vi "Periodic Tasks.vi"(8 "error in":errorcluster) -> ()   [LabVIEW 2017]
doc: "This VI runs in parallel to other tasks. It can contain as many user-defined periodic loops as you need. These can carry out PID or other sorts of timed response."
uses:
  <vilib>/Rock Robotics/WPI/ThirdParty/Phoenix-LabVIEW/Motor Controller/Controls/CTRE_Phoenix_MotorControl_FeedbackDevice.ctl
  CommandTypes/DriveCommands.ctl
  <userlib>/836-Library/Drive/Drive_Code_V2/Drive_Code_Support/PidClusters/Drive_Code_PID_Bundle.ctl
  <vilib>/Platform/TimedLoop/XDataNode/timing_clust.ctl
  <vilib>/Platform/TimedLoop/XDataNode/nitl_modes.ctl
  <vilib>/Platform/TimedLoop/XDataNode/wakeup.ctl
  <userlib>/836-Library/Drive/Drive_Code_V2/Drive_Code_Support/SensorTypedefs/Sensor_Cluster.ctl
  <userlib>/836-Library/Drive/Drive_Code_V2/Drive_Code_Support/SensorTypedefs/Camera_Cluster.ctl
  <vilib>/Rock Robotics/WPI/RobotDrive/WPI_RobotDriveDevRef.ctl
  <vilib>/Rock Robotics/WPI/MotorControl/WPI_MotorControlDeviceRef.ctl
  <vilib>/Rock Robotics/WPI/MotorControl/WPI_MotorControlType.ctl
  <vilib>/Rock Robotics/SystemInterfaces/DIO/FPGA_DIOPWMChannel.ctl
  <vilib>/Rock Robotics/WPI/PWM/WPI_PWMDeadband.ctl
  <vilib>/Rock Robotics/SystemInterfaces/DIO/FPGA_DIOChannel.ctl
  <userlib>/836-Library/Drive/Drive_Code_V2/Drive_Code_Support/DriveTrains/Drive_Trains.ctl
  <userlib>/836-Library/Drive/Drive_Code_V2/Drive_Code_Support/Command_Sends/Drive_Code_Command_Type.ctl
  <userlib>/836-Library/Drive/Drive_Code_V2/Drive_Code_Support/Command_Sends/Drive_Code_Command_List.ctl
  <userlib>/836-Library/Drive/Drive_Code_V2/Drive_Code_Support/PidClusters/PidInversions.ctl
  <userlib>/836-Library/Drive/Drive_Code_V2/Drive_Code_Support/PidClusters/DrivePidInputs.ctl
  <userlib>/836-Library/Drive/Drive_Code_V2/Drive_Code_Support/PidClusters/PidInputs.ctl
  <userlib>/836-Library/Drive/Drive_Code_V2/Drive_Code_Support/Command_Sends/Command_Tolerances.ctl
  <userlib>/836-Library/Drive/Drive_Code_V2/Drive_Code_Support/Command_Sends/Command_Tolerance_Info.ctl
  <userlib>/836-Library/System/QCP_V2/QCPSupportCode/QCPData.ctl
  <vilib>/Rock Robotics/WPI/Relay/WPI_RelayValue.ctl
  <vilib>/Rock Robotics/WPI/DriverStation/WPI_DriverStationRobotMode2.ctl
  <userlib>/836-Library/Drive/Drive_Code_V2/Drive_Code_Support/CmdFinishedTypes.ctl
  <vilib>/Rock Robotics/WPI/ThirdParty/Phoenix-LabVIEW/Motor Controller/Get/CTRE_Phoenix_MotorController_GetPulseWidthAll.vi
  <vilib>/Rock Robotics/Network Tables/NT Read Number.vi
  <vilib>/Rock Robotics/Network Tables/NT Write Number.vi
  <userlib>/836-Library/Drive/Drive_Code_V2/Drive_Code_Support/Command_Sends/Drive_Cmd_PID_Update.vi
  <userlib>/836-Library/Drive/Drive_Code_V2/Drive_Code_Support/Command_Sends/Drive_Cmd_Follow_Camera.vi
  <userlib>/836-Library/Drive/Drive_Code_V2/Drive_Code_Support/Command_Sends/Drive_Cmd_Turn_to_Camera.vi
  <vilib>/addons/control/pid/pid.llb/PID Output Rate Limiter (DBL).vi
  <userlib>/836-Library/Drive/Drive_Code_V2/Drive_Code_Support/Command_Sends/Drive_Cmd_Cheesey_Drive.vi
  <vilib>/platform/TimedLoop/XDataNode/XDataNode.xnode
  <vilib>/Platform/TimedLoop/XDataNode/XDNodeRunTimeDep.lvlib
  <vilib>/addons/control/pid/NI_PID_pid.lvlib
  <vilib>/Rock Robotics/WPI/Power/WPI_Power Get 5Volt Rail Voltage and Current.vi
panel:
  in  "Tab Control":T1(tab)=enum."Sensors"
  out "SensorsFinished Late? [i-1]":bool=TRUE
  out "SensorsIterationDuration":i64=26
  out "QCP Finished Late? [i-1]":bool
  out "QCP Iteration Duration":i64=3
  in  "SensorPeriod":i64=20
  in  "QCPPeriod":i64=20
  out "DriveFinished Late? [i-1]":bool
  out "Drive Iteration Duration":i64=4
  in  "Drive Period":i64=40
  out "PID Finished Late? [i-1]":bool
  out "PID Iteration Duration":i64
  in  "PIDPeriod":i64=400
  out "Intake Iteration Duration":i64
  out "Intake Finished Late? [i-1]":bool
  in  "Intake Period":i64=50
  out "Lift Finished Late? [i-1]":bool=TRUE
  out "Lift Iteration Duration":i64=25
  in  "Lift Period":i64=20
  out "Lift_Command":T2(ring)=enum."Home"
  in  "Verticle_Mech_Hi":dbl
  in  "Verticle_Mech_Low":dbl=24.1875
  in  "Verticle_Sensor_Low":dbl=587.0
  in  "Rotation_Mech_Low":dbl=90.0
  in  "Verticle_Sensor_Hi":dbl=26537.0
  in  "Rotation_Mech_Hi":dbl
  in  "Rotation_Sensor_Low":dbl=6193.0
  in  "Rotation_Sensor_Hi":dbl=894.0
  in  "Position":dbl(knob) scale=0.0..1.0
  in  "Intake Speed":dbl(knob)=0.7699909222498021 scale=0.0..1.0
  out "Intake_Command":T3(ring)
  in  "Cube? Fakeout":bool=TRUE
  out "Cube?":bool=TRUE
  out "Steer Fed Value":dbl(graph)
  out "Dist Resp":cluster{"Setpoint":dbl, "Process":dbl}(graph)
  out "Angle Resp":cluster{"Setpoint":dbl, "Process":dbl}(graph)
  in  "Steer Scale":dbl(knob)=0.500001840510888 scale=0.0..1.0
  in  "Turn In Place Deadband":dbl(knob)=0.12768422674403432 scale=0.0..0.4
  in  "Throttle Scale":dbl(knob)=1.0 scale=0.0..1.0
  in  "Square Wheel":bool=TRUE
  in  "Square Throttle":bool=TRUE
  in  "Update PID":bool
  in  "AquireSpeed":dbl(knob) scale=0.0..10.0
  in  "CenterOnCubeTolerance":dbl=0.5
  in  "CenterSpeed":dbl(knob) scale=0.0..1.0
  in  "Yaw_Holding_Still_PID_Gains":T4={"proportional gain (Kc)"=0.021, "integral time (Ti, min)"=0.0, "derivative time (Td, min)"=0.0} {"derivative time (Td, min)" format="%.3f"; "integral time (Ti, min)" format="%.3f"; "proportional gain (Kc)" format="%.3f"}
  in  "Distance_Holding_Still_PID_gains":T4={"proportional gain (Kc)"=0.025, "integral time (Ti, min)"=0.013, "derivative time (Td, min)"=0.003} {"derivative time (Td, min)" format="%.3f"; "integral time (Ti, min)" format="%.3f"; "proportional gain (Kc)" format="%.3f"}
  in  "Distance_Driving_Straight_PID_Gains":T4={"proportional gain (Kc)"=0.025, "integral time (Ti, min)"=0.0125, "derivative time (Td, min)"=0.0025} {"derivative time (Td, min)" format="%.3f"; "integral time (Ti, min)" format="%.3f"; "proportional gain (Kc)" format="%.3f"}
  in  "Yaw_Driving_Straight_PID_gains":T4={"proportional gain (Kc)"=0.021, "integral time (Ti, min)"=0.0, "derivative time (Td, min)"=0.0} {"derivative time (Td, min)" format="%.3f"; "integral time (Ti, min)" format="%.3f"; "proportional gain (Kc)" format="%.3f"}
  out "Drive Command":T5(ring)=enum."Manual"
  in  "Acceleration Throttle Rate Limit":dbl(knob)=208.87815423820334 scale=200.0..400.0
  in  "Acceleration Steer Rate Limit":dbl(knob)=1540.1240783536919 scale=50.0..5000.0
  in  "Throttle Slow Mode Mult":dbl(knob)=0.518053304835497 scale=0.0..1.0
  in  "Steer Slow Mode Mult":dbl(knob)=0.5622816498580822 scale=0.0..1.0
  in  "Deceleration Steer Rate Limit":dbl(knob)=1e+27 scale=50.0..1e+27
  in  "DecelerationThrottle Rate Limit":dbl(knob)=1498.2967839773426 scale=200.0..1500.0
  in  "Read Drive QCP":bool
  in  "Read Lift QCP":bool
  in  "Read Auto QCP":bool
  in  "Read Intake QCP":bool
  in  "Read Sensor QCP":bool
  in  "DriveWriteQCPFile":bool
  in  "DriveTuningMode?":bool=TRUE
  in  "LiftWriteQCPFile":bool
  in  "LiftTuningMode?":bool=TRUE
  in  "AutoWriteQCPFile":bool
  in  "AutoTuningMode?":bool
  in  "IntakeWriteQCPFile":bool
  in  "IntakeTuningMode?":bool=TRUE
  in  "SensorWriteQCPFile":bool
  in  "SensorTuningMode?":bool
  out "Right Encoder":dbl(graph)=1039.4189824999999
  out "Left Encoder":dbl(graph)
  in  "PBot Lift Pitch Ref":dbl=230.0
  in  "Reset Lift Rate":bool
  out "IMU Rate Lift":dbl
  out "IMU Lift Max Rate":dbl
  out "IMU LIft Rate":dbl(graph)
  in  "Lift Is IMU?":bool
  out "Pitch  Drive":dbl(graph)
  out "Roll Drive":dbl(graph)
  out "Yaw Drive":dbl(graph)
  out "RightDriveEncoder":dbl=1039.4189824999999
  out "Cube? 4":bool
  out "LeftDriveEncoder":dbl=801.3391574999999
  out "LiftElevation":dbl=-21.72307803468208
  out "LiftRotation":dbl=-14.878278920551049
  out "Cube? 3":bool
  out "Cube? 5":bool
  out "Cube? 6":bool
  out "Cube? 1":bool
  out "Cube? 2":bool
  out "Yaw Wind Drive":dbl
  out "Roll Wind Drive":dbl
  out "Pitch Wind Drive":dbl
  out "Valid Target":bool
  out "tx":dbl
  in  "ledMode":dbl=1.0
  in  "pipeline":dbl
  in  "userMode":dbl
  in  "Restart Limelight":bool
  out "Yaw Wind LiftArm":dbl
  out "Roll WindLiftArm":dbl
  out "Pitch LiftArm":dbl=-87.0
  out "YawLiftArm":dbl(graph)
  out "Roll LiftArm":dbl(graph)
  out "Pitch LiftArm":dbl(graph)
  out "Raw Lift Elevation":i32=3231
  out "Raw Lift Rotation":i32=1770
  in  "Lift Pitch Ref":dbl=87.0
  out "Lift IMU Fault":bool
  in  "Hyster":dbl=0.3
  in  "Rate Thresh":dbl=500.0 step=0.001
  in  "hi limit":dbl=35.0
  in  "lo limit":dbl=-211.0
  out "Total Current (A)":dbl
  out "Current (A)":dbl
  in  "Reet Max Total":bool
  out "Max Total Current":dbl=282.75
  out "PDP Total Current":dbl(graph)
  in  "Reset Max Current?":bool
  out "Max Current (A)":dbl
  in  "PDP Channel":dbl=10.0
  out "PDP Channel Current (A)":dbl(graph)
  out "Input Voltage Brown Out":bool
  out "3.3V User Rail Short":bool
  out "5 V User Rail Short":bool
  out "6 V User Rail Short":bool
  out "5V User Rail Brown Out":bool
  out "5 volt rail voltage (V)":dbl=4.950481445312501
  out "5 volt rail current (A)":dbl=0.289408203125
  in  "Reset Voltage Max":bool
  out "Voltage Min":dbl=4.949025878906251
  in  "Reset Current Max":bool
  out "5V Rail Current Max":dbl=0.289408203125
  in  "Current Tolerance":dbl=100.0
  in  "Current Limit?":bool=TRUE
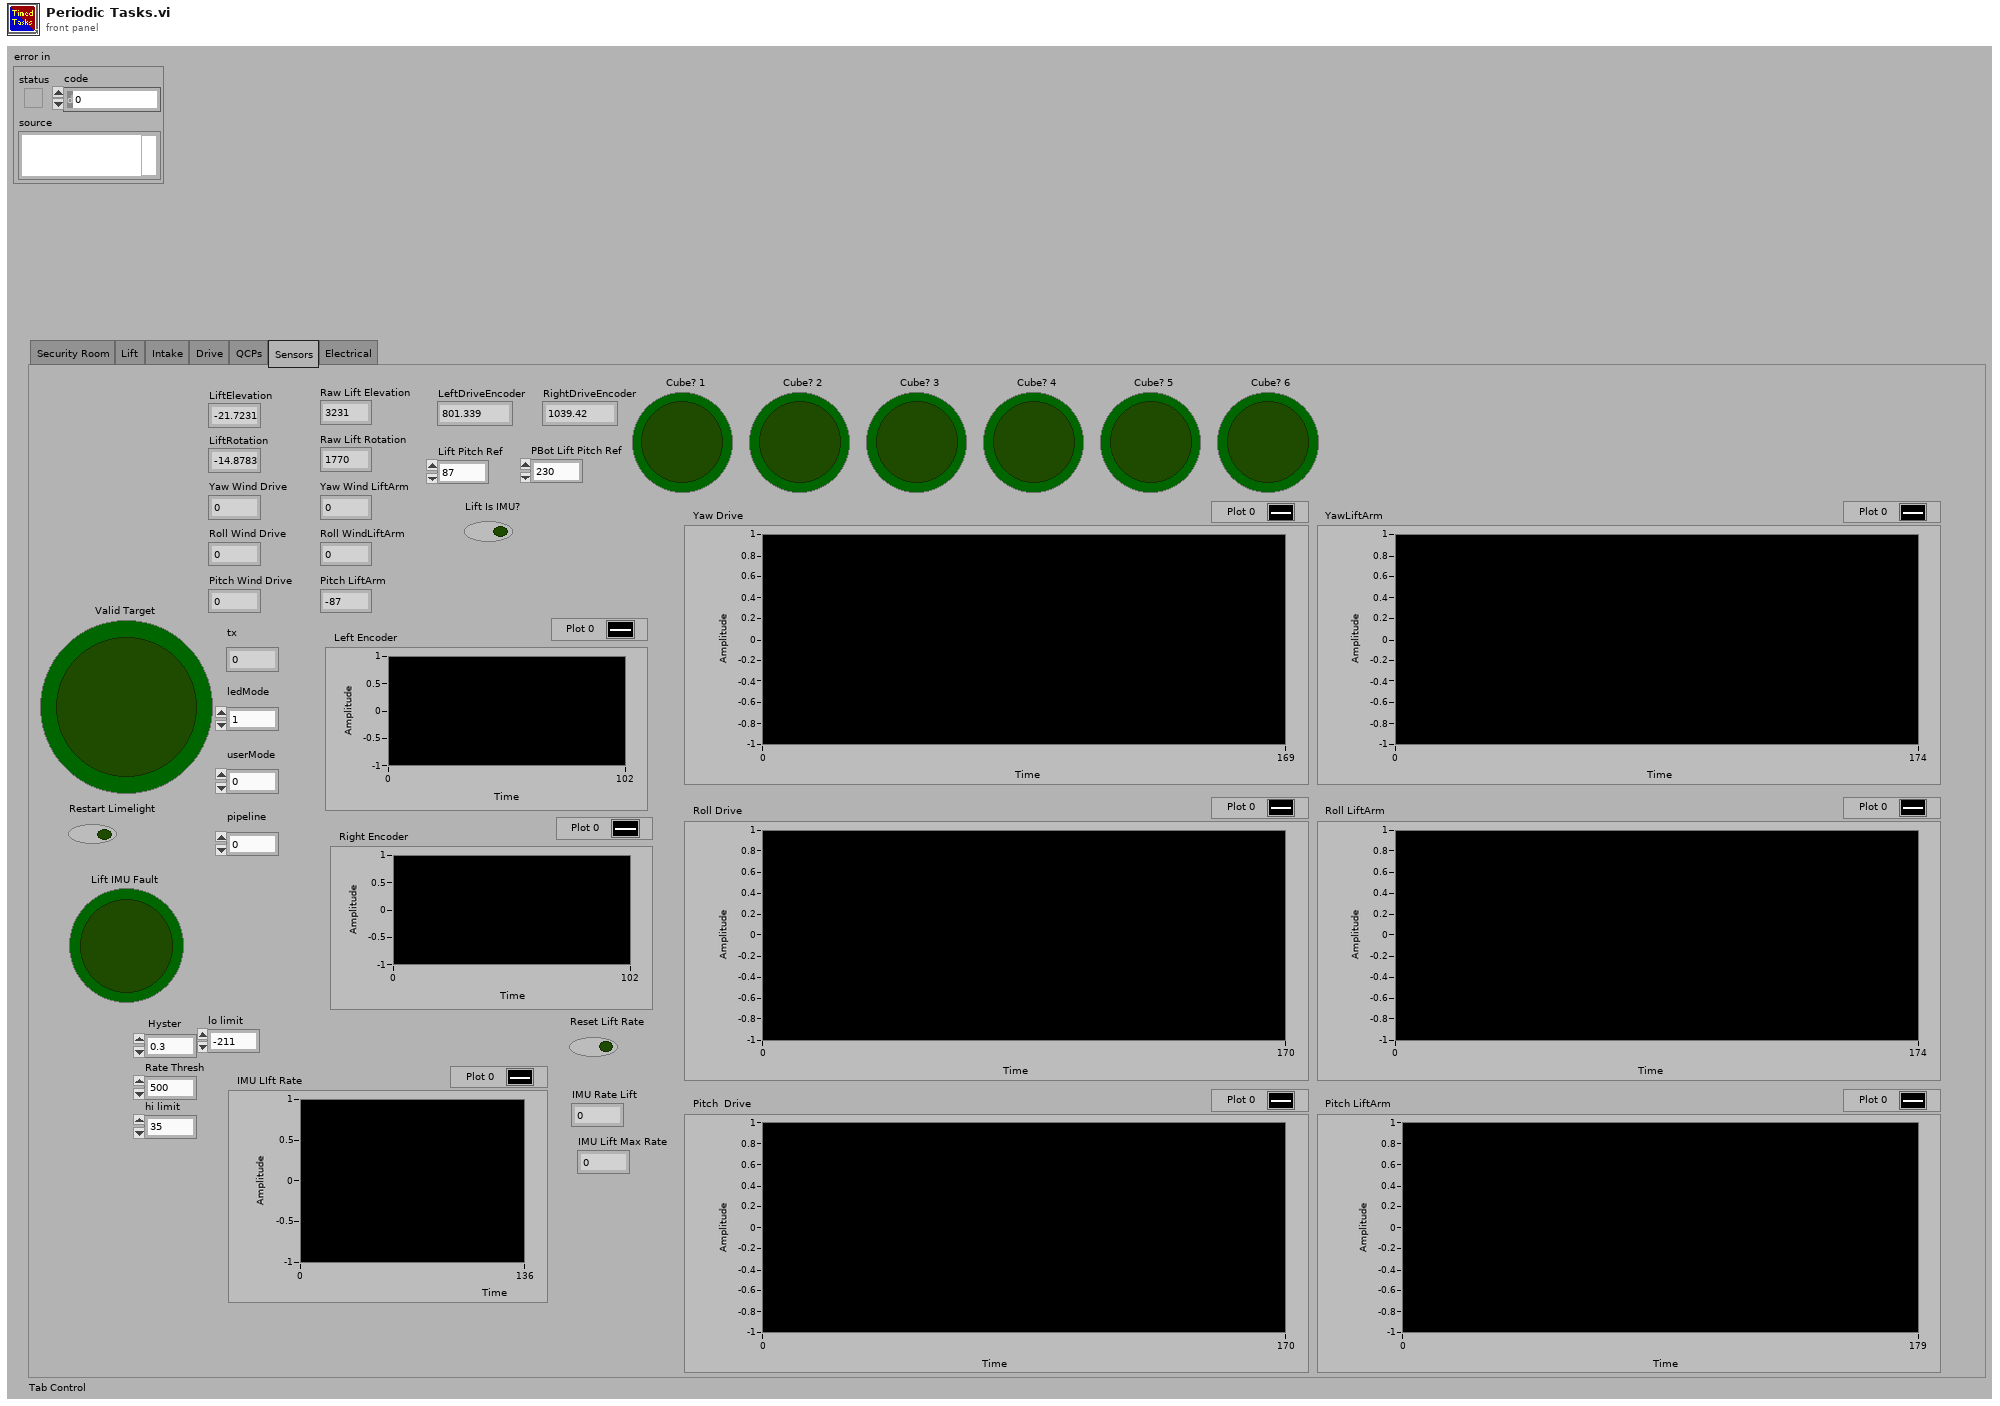
[diagram p1: front panel]
types:
  T1 = enum32{"Security Room", "Lift", "Intake", "Drive", "QCPs", "Sensors", "Electrical"}
  T2 = enum16{"Do  Nothing", "Manuel", "Home", "Ground", "To Switch", "To Scale Low", "To Scale Medium", "To Scale High"}
  T3 = enum16{"Do Nothing", "Manuel", "Score", "Acquire"}
  T4 = cluster{"proportional gain (Kc)":dbl, "integral time (Ti, min)":dbl, "derivative time (Td, min)":dbl}
  T5 = enum16{"Center on Cube", "Manual", "Acquire Cube", "Drive Path"}
  T6 = typedef "Drive_Code_PID_Bundle.ctl" = cluster{"Yaw, Driving Straight":cluster{"proportional gain (Kc)":dbl, "integral time (Ti, min)":dbl, "derivative time (Td, min)":dbl}, "Yaw, Holding Still":cluster{"proportional gain (Kc)":dbl, "integral time (Ti, min)":dbl, "derivative time (Td, min)":dbl}, "Distance, Driving Straight":cluster{"proportional gain (Kc)":dbl, "integral time (Ti, min)":dbl, "derivative time (Td, min)":dbl}, "Distance, Holding Still":cluster{"proportional gain (Kc)":dbl, "integral time (Ti, min)":dbl, "derivative time (Td, min)":dbl}}
  T7 = typedef "DriveCommands.ctl" = enum16{"Center on Cube", "Manual", "Acquire Cube", "Drive Path"}
  T8 = typedef "CTRE_Phoenix_MotorControl_FeedbackDevice.ctl" = i8
  T9 = typedef "WPI_MotorControlDeviceRef.ctl" = cluster{"DeviceStatus":errorcluster, "Type":T10, "PWM":cluster{"PWM Channel":T11, "DeadBand":T12}, "CAN":cluster{"Device Number":u8, "SetOutput VI Ref":variant, "GetOutput VI Ref":variant, "Enable VI Ref":variant, "Disable VI Ref":variant, "Data":variant}, "Invert":bool, "DIO PWM":cluster{"PWM \"Enable\" Channel":T11, "DIOChannel":T13, "PWM Rate":dbl}}
  T10 = typedef "WPI_MotorControlType.ctl" = enum16{"PWM", "CAN", "DIO PWM"}
  T11 = typedef "FPGA_DIOPWMChannel.ctl" = enum8{"PWM 0", "PWM 1", "PWM 2", "PWM 3", "PWM 4", "PWM 5", "PWM 6", "PWM 7", "PWM 8", "PWM 9", "PWM MXP 0", "PWM MXP 1", "PWM MXP 2", "PWM MXP 3", "PWM MXP 4", "PWM MXP 5", "PWM MXP 6", "PWM MXP 7", "PWM MXP 8", "PWM MXP 9", "Invalid"}
  T12 = typedef "WPI_PWMDeadband.ctl" = cluster{"Name":string, "maxPositivePwm":i32, "minPositivePwm":i32, "centerPwm":i32, "maxNegativePwm":i32, "minNegativePwm":i32, "angularRange":u16}
  T13 = typedef "FPGA_DIOChannel.ctl" = enum8{"DIO 0", "DIO 1", "DIO 2", "DIO 3", "DIO 4", "DIO 5", "DIO 6", "DIO 7", "DIO 8", "DIO 9", "DIO MXP 0", "DIO MXP 1", "DIO MXP 2", "DIO MXP 3", "DIO MXP 4", "DIO MXP 5", "DIO MXP 6", "DIO MXP 7", "DIO MXP 8", "DIO MXP 9", "DIO MXP 10", "DIO MXP 11", "DIO MXP 12", "DIO MXP 13", "DIO MXP 14", "DIO MXP 15", "SPI Port CS1", "SPI Port CS2", "SPI Port CS3", "SPI Port MISO", "SPI Port MOSI", "Invalid"}
  T14 = typedef "WPI_DigitalInputDevRef.ctl" = cluster{"DevStatus":errorcluster, "DIO Channel":T13}
  T15 = typedef "XDNodeRunTimeDep.lvlib/timing_clust.ctl" = cluster{"Expected End [f-1]":u64, "Actual End [f-1]":u64, "Finished Late? [f-1]":bool, "Expected End [i-1]":u64, "Actual End [i-1]":u64, "Finished Late? [i-1]":bool, "Expected Start [i]":u64, "Actual Start [i]":u64, "Expected Start [f]":u64, "Actual Start [f]":u64, "Source Name":string, "Structure Name":string, "Period":i64, "Deadline":i64, "Offset":i64, "Start":i64, "Priority":i32, "Timeout":i32, "Mode":T16, "Wakeup Reason":T17, "Error":errorcluster, "Source Type":string, "Secondary Source Type":string, "Global End Time":u64, "Global Start Time":u64, "Frame Duration":u64, "Iteration Duration":u64, "Assigned CPU":i32, "I/O Scan Engine Mode":u32}
  T16 = typedef "XDNodeRunTimeDep.lvlib/nitl_modes.ctl" = enum32{"No Change", "Process missed periods, maintain original phase", "Discard missed periods, maintain original phase", "Process missed periods, ignore original phase", "Discard missed periods, ignore original phase"}
  T17 = typedef "XDNodeRunTimeDep.lvlib/wakeup.ctl" = enum32{"Normal", "Aborted", "Asynchronous wakeup", "Timing source error", "Timed loop error", "Timeout"}
  T18 = typedef "WPI_EncoderDevRef.ctl" = cluster{"DevStatus":errorcluster, "EncoderIndex":T19, "CounterIndex":T20, "DistancePerCount":dbl, "Decoding Type":T21}
  T19 = typedef "FPGA_EncoderIdx.ctl" = enum8{"Enc 0", "Enc 1", "Enc 2", "Enc 3", "Enc 4", "Enc 5", "Enc 6", "Enc 7", "Invalid"}
  T20 = typedef "FPGA_CounterCtrSystemIndex.ctl" = enum8{"Ctr 0", "Ctr 1", "Ctr 2", "Ctr 3", "Ctr 4", "Ctr 5", "Ctr 6", "Ctr 7", "Invalid"}
  T21 = typedef "WPI_EncoderType.ctl" = enum16{"1x", "2x", "4x"}
  T22 = typedef "ImuDevRef.ctl" = cluster{"I2CDevRef":T23, "Valid Cal File?":bool}
  T23 = typedef "WPI_I2CDevRef.ctl" = cluster{"DevStatus":errorcluster, "Device Address":u8, "Handle":i32, "I2C Bus":T24}
  T24 = typedef "i2c_bus.ctl" = enum16{"I2C On-Board", "I2C MXP", "Invalid"}
  T25 = typedef "WPI_RelayDevRef.ctl" = cluster{"DevStatus":errorcluster, "Relay Channel":T26, "Relay Direction":T27}
  T26 = typedef "FPGA_DIORelayChannel.ctl" = enum8{"Relay 0", "Relay 1", "Relay 2", "Relay 3", "Invalid"}
  T27 = typedef "WPI_RelayDirection.ctl" = enum16{"Both directions", "Forward only", "Reverse only"}
  T28 = typedef "WPI_RelayValue.ctl" = enum16{"Off", "On", "Forward", "Reverse"}
  T29 = enum16{"[0, 360]", "[-180, 180]", "[0, 2PI]", "[-PI, PI]"}
  T30 = cluster{"Yaw":dbl, "Roll":dbl, "Pitch":dbl, "Yaw Wind":dbl, "Roll Wind":dbl, "Pitch Wind":dbl}
  T31 = typedef "Sensor_Cluster.ctl" = cluster{"Gyro Data":cluster{"Gyro RT FIFO":refnum<k33>, "Gyro Current":dbl, "Gyro Hold":dbl}, "Encoder Data":cluster{"Encoder RT FIFO":refnum<k33>, "Encoder Current":dbl, "Encoder Hold":dbl}, "Camera Data":cluster{"Camera RT FIFO":refnum<k33>, "Camera Current":T32}}
  T32 = typedef "Camera_Cluster.ctl" = cluster{" Angle":dbl, "Valid":bool}
  T33 = typedef "WPI_RobotDriveDevRef.ctl" = cluster{"DevStatus":errorcluster, "Motors[]":T9[], "Square Inputs":bool, "Max Output":dbl}
  T34 = typedef "Drive_Trains.ctl" = enum16{"Tank Drive 2 Motor", "Tank Drive 4 Motor", "Tank Drive 6 Motor", "Mecanum Drive", "Kiwi Drive", "Invalid"}
  T35 = typedef "PidInversions.ctl" = cluster{"Distance PID Inverted?":bool, "Yaw PID Inverted?":bool}
  T36 = cluster{"Cluster":T31, "RobotDriveDevRef":T33, "Enum":T34, "Valid Commands":bool[], "Drive Comand Notifier":refnum<notifier>, "Command Finished?":refnum<k4>, "Command Canceled":refnum<k4>, "PID Inversions":T35, "PID Inputs Notifier":refnum<notifier>, "Cmd Tol Notifier":refnum<notifier>}
  T37 = typedef "Semaphore RefNum" = refnum<k1>
  T38 = cluster{"Data Value Refnum":refnum<data-value>, "semaphore":T37}
  T39 = typedef "QCP_RefNum.ctl" = cluster{"Data Value Refnum":refnum<data-value>, "semaphore":T37}
  T40 = typedef "WPI_ServoDeviceRef.ctl" = cluster{"DeviceStatus":errorcluster, "PWM Channel":T11, "DeadBand":T12}
  T41 = typedef "Command_Tolerances.ctl" = cluster{"Distance":T42, "Yaw":T42}
  T42 = typedef "Command_Tolerance_Info.ctl" = cluster{"Upper Error Bound":dbl, "Lower Error Bound":dbl}
  T43 = typedef "WPI_DriverStationRobotMode2.ctl" = enum16{"Autonomous Disabled", "Autonomous Enabled", "Teleop Disabled", "Teleop Enabled", "Disconnected", "Finish", "Test Disabled", "Test Enabled", "Emergency Stopped"}
  T44 = typedef "CmdFinishedTypes.ctl" = enum16{"Poll", "Blocking"}
  T45 = typedef "DrivePidInputs.ctl" = cluster{"EncoderPID":T46, "YawPID":T46}
  T46 = typedef "PidInputs.ctl" = cluster{"Setpoint":dbl, "Process":dbl}
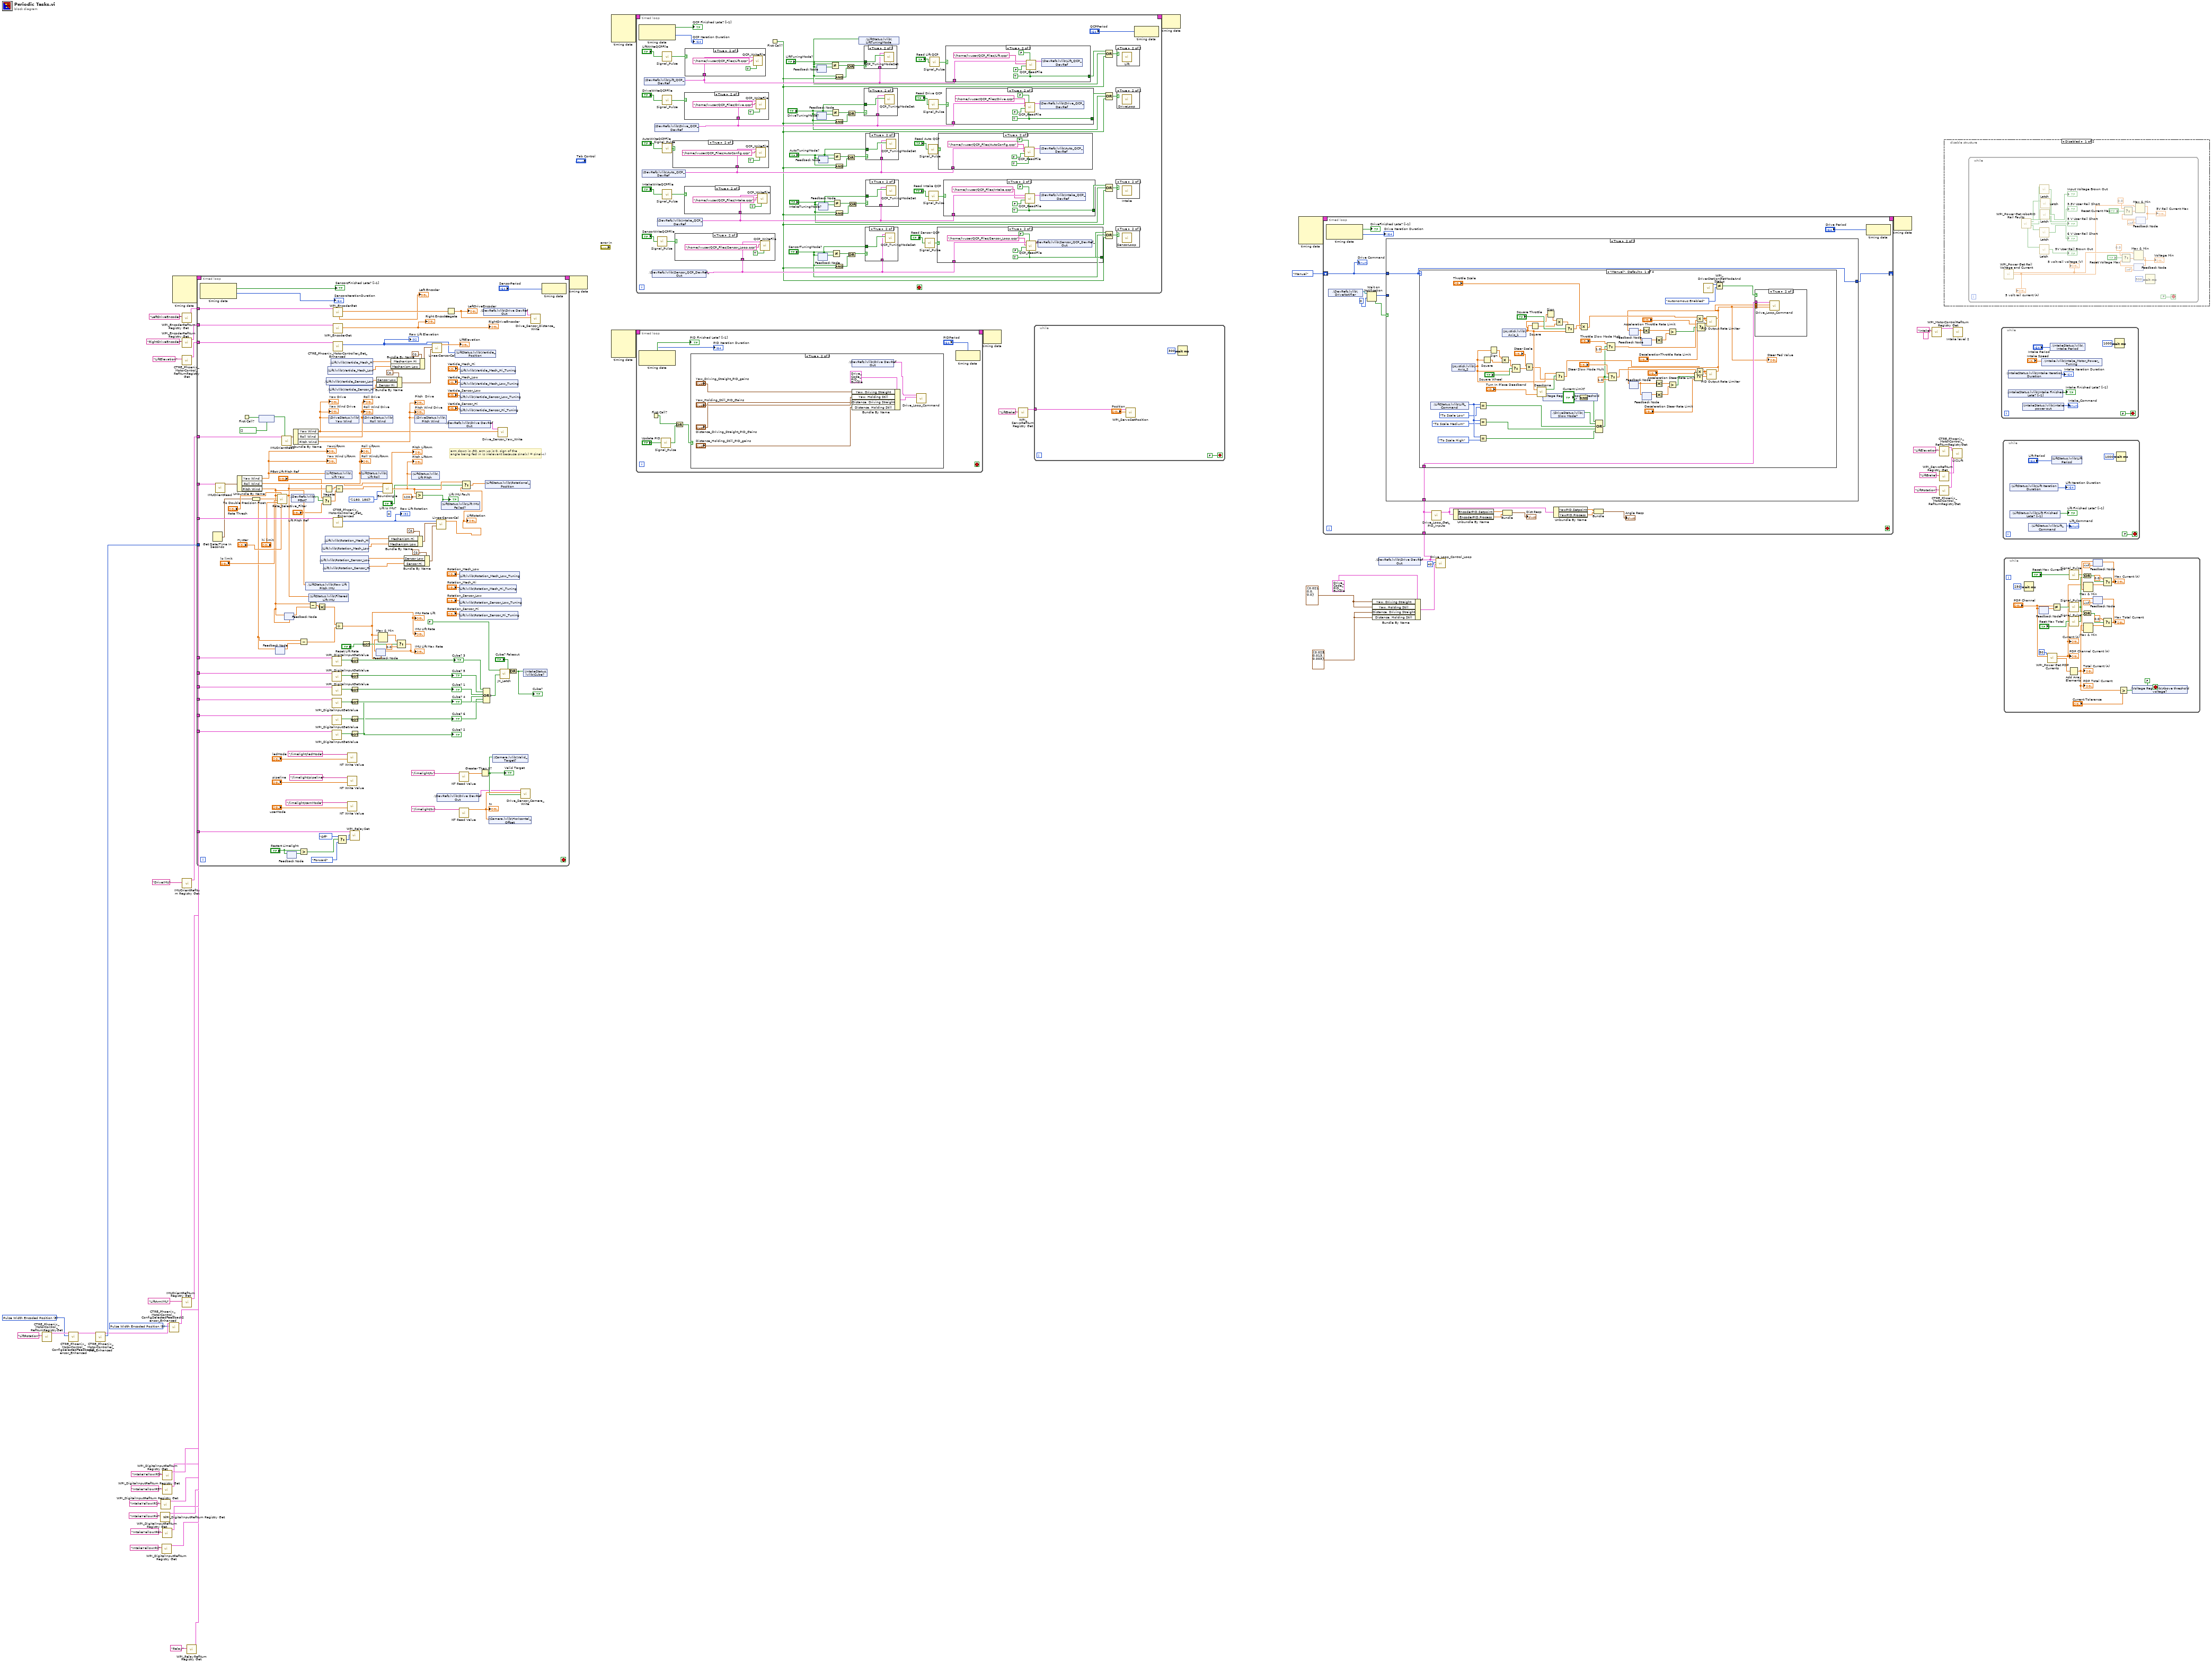
[diagram p0: block diagram]
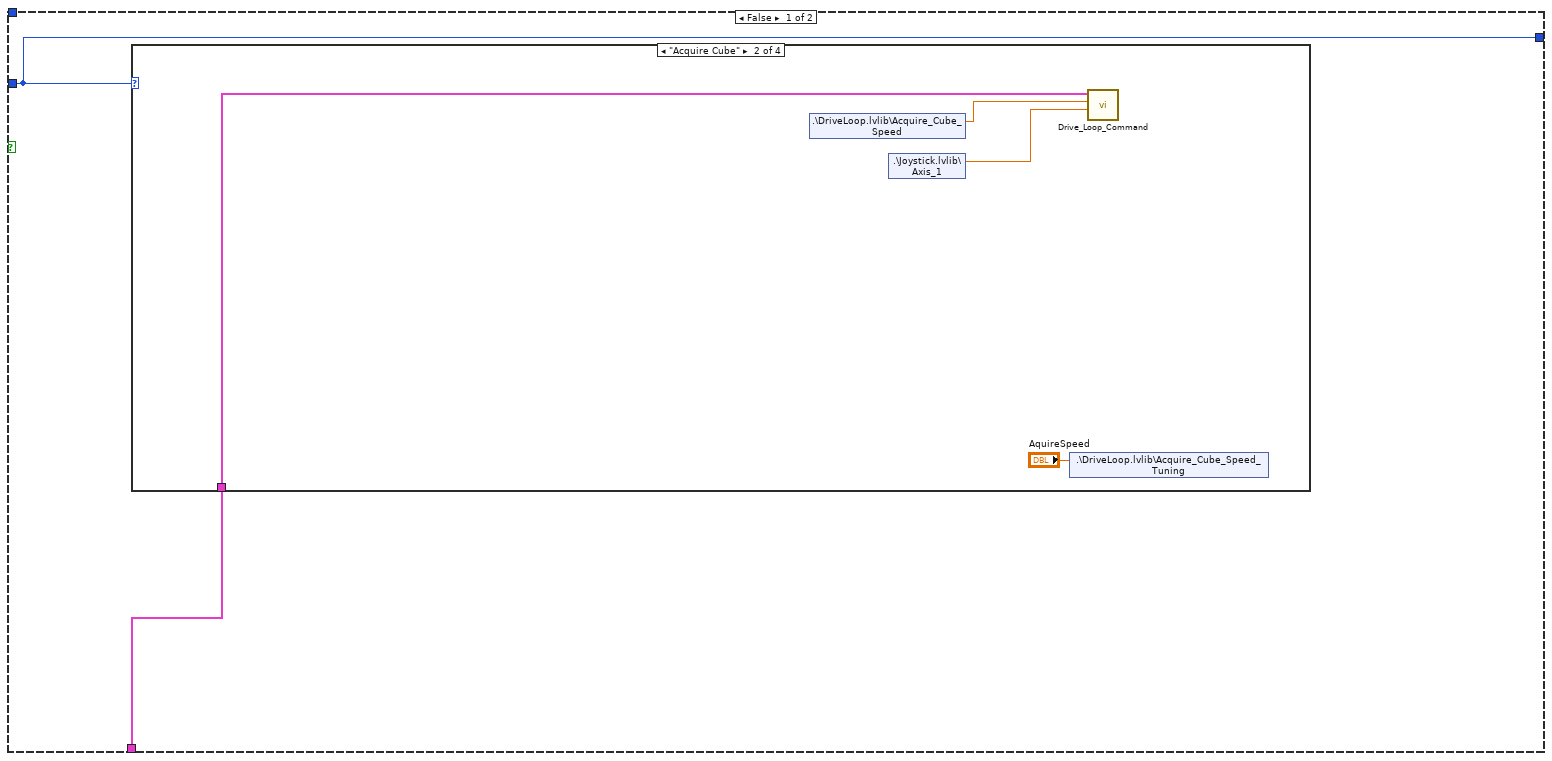
[diagram p2: hidden frame]
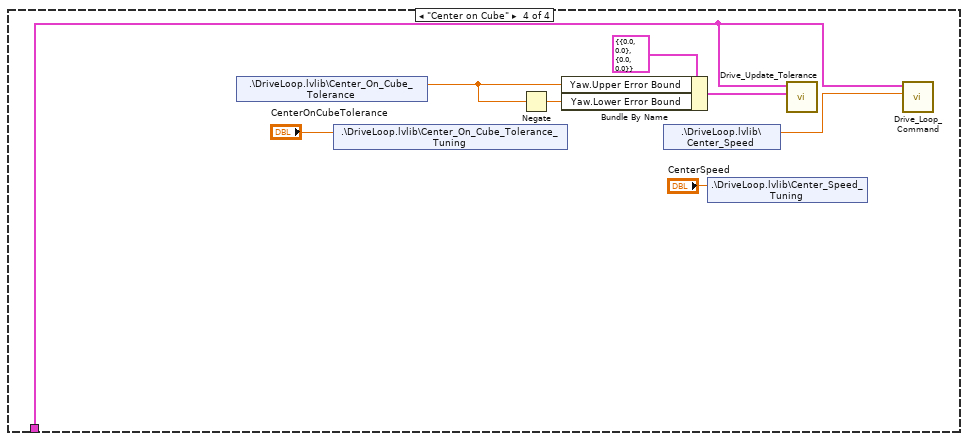
[diagram p5: hidden frame]
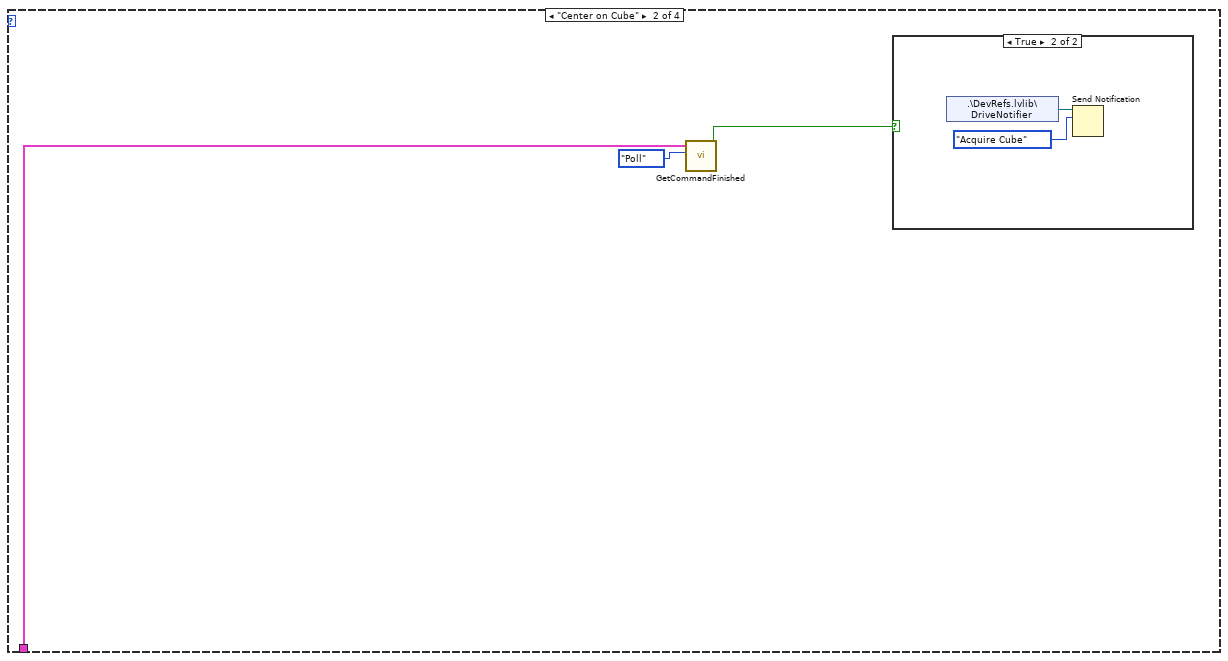
[diagram p7: hidden frame]
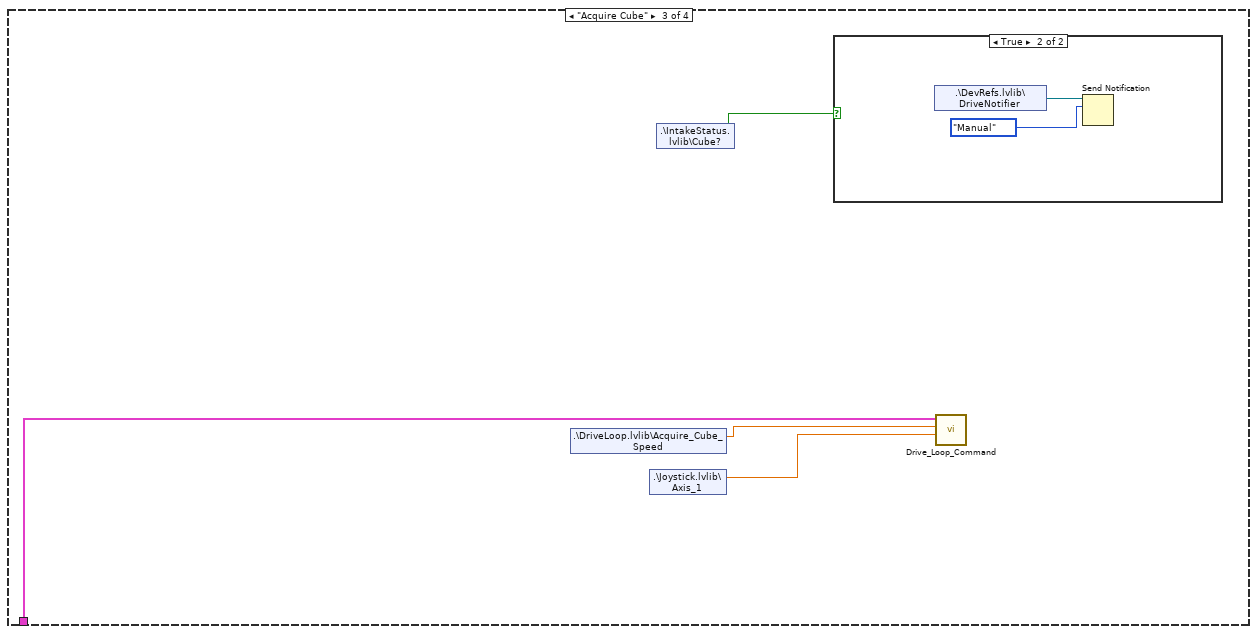
[diagram p9: hidden frame]
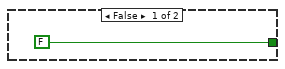
[diagram p17: hidden frame]
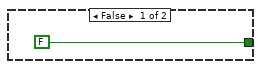
[diagram p18: hidden frame]
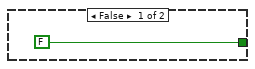
[diagram p20: hidden frame]
diagram:
  w4 = T4 {"proportional gain (Kc)"=0.025, "integral time (Ti, min)"=0.013, "derivative time (Td, min)"=0.003} ("Distance, Driving Straight")
  w5 = T4 {"proportional gain (Kc)"=0.021, "integral time (Ti, min)"=0.0, "derivative time (Td, min)"=0.0} ("Yaw, Driving Straight")
  w35 = T8 8 items=["None"=-1, "QuadEncoder"=0, "Analog"=2, "Tachometer"=4, "Pulse Width Encoded Position"=8, "Sensor Sum (S0 + S1)"=9, "Sensor Difference (D0 - D1)"=10, "Remote Source 0"=11, "Remote Source 1"=12, "Software Emulated"=15] ("Feedback Device")
  w39 = T8 8 items=["None"=-1, "QuadEncoder"=0, "Analog"=2, "Tachometer"=4, "Pulse Width Encoded Position"=8, "Sensor Sum (S0 + S1)"=9, "Sensor Difference (D0 - D1)"=10, "Remote Source 0"=11, "Remote Source 1"=12, "Software Emulated"=15] ("Feedback Device")
  n1 = call <vilib>:"CTRE_Phoenix_MotorControl_RefNumRegistryGet.vi"("refnum name"="LiftRotation") -> ("PhoenixMotorControlDevRef"=w40:T9)  [unwired: 9 in, 1 out]
  n2 = call <vilib>:"CTRE_Phoenix_MotorControl_ConfigSelectedFeedbackSensor_Enhanced.vi"("Feedback Device"=w39, "PhoenixMotorControlDevRef"=w40) -> ("PhoenixMotorControlDevRef"=w38:T9)  [unwired: 8 in, 1 out]
  n3 = call-poly <vilib>:"CTRE_Phoenix_MotorController_Get_Enhanced.vi"("PhoenixMotorControlDevRef"=w38) -> ("PhoenixMotorControlDevRef"=w36:T9, "Pulse Width Position"=w37:i32)  [unwired: 9 in, 4 out]
  n4 = call <vilib>:"WPI_DigitalInputRefNum Registry Get.vi"("refnum name"="IntakeYellowIR4") -> ("DigitalInputDevRef"=w55:T14)  [unwired: 9 in, 1 out]
  n5 = call <vilib>:"WPI_DigitalInputRefNum Registry Get.vi"("refnum name"="IntakeYellowIR1") -> ("DigitalInputDevRef"=w46:T14)  [unwired: 9 in, 1 out]
  n6 = call <vilib>:"WPI_DigitalInputRefNum Registry Get.vi"("refnum name"="IntakeYellowIR2") -> ("DigitalInputDevRef"=w45:T14)  [unwired: 9 in, 1 out]
  n7 = call <vilib>:"WPI_DigitalInputRefNum Registry Get.vi"("refnum name"="IntakeYellowIR5") -> ("DigitalInputDevRef"=w48:T14)  [unwired: 9 in, 1 out]
  n8 = call <vilib>:"WPI_DigitalInputRefNum Registry Get.vi"("refnum name"="IntakeYellowIR6") -> ("DigitalInputDevRef"=w47:T14)  [unwired: 9 in, 1 out]
  n9 = call <vilib>:"WPI_DigitalInputRefNum Registry Get.vi"("refnum name"="IntakeYellowIR3") -> ("DigitalInputDevRef"=w53:T14)  [unwired: 9 in, 1 out]
  n10 = call <vilib>:"CTRE_Phoenix_MotorControl_ConfigSelectedFeedbackSensor_Enhanced.vi"("Feedback Device"=w35, "PhoenixMotorControlDevRef"=w36) -> ("PhoenixMotorControlDevRef"=w34:T9)  [unwired: 8 in, 1 out]
  n11 = node-c288() -> (w31:T15)  [unwired: 4 in]
  n12 = call <vilib>:"WPI_EncoderRefNum Registry Get.vi"("refnum name"="LeftDriveEncoder") -> ("EncoderDevRef"=w22:T18)  [unwired: 9 in, 1 out]
  n13 = call <vilib>:"WPI_EncoderRefNum Registry Get.vi"("refnum name"="RightDriveEncoder") -> ("EncoderDevRef"=w23:T18)  [unwired: 9 in, 1 out]
  n14 = call <vilib>:"CTRE_Phoenix_MotorControl_RefNumRegistryGet.vi"("refnum name"="LiftElevation") -> ("PhoenixMotorControlDevRef"=w24:T9)  [unwired: 9 in, 1 out]
  n15 = call <userlib>:"IMUOrientRefNum Registry Get.vi"("refnum name"="DriveIMU") -> ("IMUDevRef out"=w28:T22)  [unwired: 9 in, 1 out]
  n16 = call <userlib>:"IMUOrientRefNum Registry Get.vi"("refnum name"="LiftArmIMU") -> ("IMUDevRef out"=w41:T22)  [unwired: 9 in, 1 out]
  n17 = call <vilib>:"WPI_RelayRefNum Registry Get.vi"("refnum name"="Relay") -> ("RelayDevRef"=w43:T25)  [unwired: 9 in, 1 out]
  n18 = timed-loop {
    timing: w31 -> [_]
    timing-out: [_] -> w30
    tunnel: w55 -> [w184]
    tunnel: w34 -> [w183]
    tunnel: w24 -> [w182]
    tunnel: w23 -> [w181]
    tunnel: w22 -> [w180]
    tunnel: w28 -> [w176]
    tunnel: w53 -> [w174]
    tunnel: w48 -> [w173]
    tunnel: w47 -> [w172]
    tunnel: w46 -> [w171]
    tunnel: w45 -> [w170]
    tunnel: w43 -> [w135]
    tunnel: w41 -> [w128]
    tunnel: w37 -> [_]
    stop <- _ stop-if-true
    (unwired) 0
    # "arm down is -90, arm up is 0. sign of the \nangle being fed in is irrelevant because sine(x) = sine(-x)"
    n19 = node-c288() -> (→"SensorsFinished Late? [i-1]":bool, →"SensorsIterationDuration":i64)  [unwired: 1 in]
    n20 = Get Date/Time In Seconds() -> (seconds since 1Jan1904=w79:timestamp)
    n21 = call <userlib>:"IMUOrientRead.vi"("IMU Dev Ref"=w128) -> ("Orient Y/R/P"=w127:T30)  [unwired: 7 in, 7 out]
    n22 = Unbundle By Name(w127) -> ("Yaw Wind"=w130:dbl, "Roll Wind"=w129:dbl, "Pitch Wind"=w77:dbl)
    "Yaw Wind LiftArm" <- w130
    "Roll WindLiftArm" <- w129
    "YawLiftArm" <- w130
    "Roll LiftArm" <- w129
    n23 = First Call?() -> (First Call?: T/F=w125:bool)
    n24 = To Double Precision Float(number=w79) -> (double precision float=w69:dbl)
    n25 = feedback #1(bool[] []) -> (w124:bool)
    n26 = feedback-in #1(w125) -> ()
    n27 = feedback-in #2(w69) -> ()
    n28 = feedback #2() -> (w68:dbl)  [unwired: 1 in]
    n29 = call <userlib>:"Rate_Selective_Filter.vi"("Hyster"="Hyster", "Rate Thresh"="Rate Thresh", "hi limit"="hi limit", "lo limit"="lo limit", "Time"=w69, "Distance"=w77) -> ("Filtered"=w80:dbl)  [unwired: 1 in, 2 out]
    "Pitch LiftArm" <- w80
    n30 = call <userlib>:"IMUOrientRead.vi"("IMU Dev Ref"=w176, "Orient Reset (Wind)"=w124) -> ("Orient Y/R/P"=w175:T30)  [unwired: 6 in, 7 out]
    n31 = feedback-in #3(w77) -> ()
    n32 = feedback #3(w77) -> (w78:dbl)
    n33 = feedback #4() -> (w89:bool)  [unwired: 1 in]
    n34 = feedback-in #4("Restart Limelight") -> ()
    n35 = shared-variable ".\\DevRefs.lvlib\\PBot?"() -> (w61:bool)  [unwired: 1 in, 1 out]
    n36 = Unbundle By Name(w175) -> ("Yaw Wind"=w115:dbl, "Roll Wind"=w154:dbl, "Pitch Wind"=w153:dbl)
    "Yaw Wind Drive" <- w115
    "Roll Wind Drive" <- w154
    "Pitch Wind Drive" <- w153
    "Yaw Drive" <- w115
    "Roll Drive" <- w154
    "Pitch  Drive" <- w153
    n37 = Subtract(x=w69, y=w68) -> (x-y=w66:dbl)
    n38 = Greater?(x="Restart Limelight", y=w89) -> (0:w90:bool)
    n39 = shared-variable ".\\LiftStatus.lvlib\\Raw Lift Pitch IMU"(w77) -> ()  [unwired: 1 in, 1 out]
    n40 = Subtract(x=w77, y=w78) -> (x-y=w76:dbl)
    n41 = shared-variable ".\\LiftStatus.lvlib\\Filtered Lift IMU"(w80) -> ()  [unwired: 1 in, 1 out]
    n42 = Absolute Value(x=w76) -> (abs(x)=w67:dbl)
    n43 = shared-variable ".\\Lift.lvlib\\Rotation_Sensor_Low"() -> (w148:dbl)  [unwired: 1 in, 1 out]
    n44 = Select(t="PBot Lift Pitch Ref", s=w61, f="Lift Pitch Ref") -> (s? t:f=w64:dbl)
    n45 = shared-variable ".\\Lift.lvlib\\Rotation_Mech_Low"() -> (w163:dbl)  [unwired: 1 in, 1 out]
    n46 = shared-variable ".\\Lift.lvlib\\Rotation_Sensor_Hi"() -> (w147:dbl)  [unwired: 1 in, 1 out]
    n47 = Negate(x=w80) -> (-x=w123:dbl)
    n48 = shared-variable ".\\LiftStatus.lvlib\\Lift Yaw"(w130) -> ()  [unwired: 1 in, 1 out]
    n49 = shared-variable ".\\Lift.lvlib\\Rotation_Mech_Hi"() -> (w149:dbl)  [unwired: 1 in, 1 out]
    n50 = shared-variable ".\\Lift.lvlib\\Verticle_Sensor_Low"() -> (w140:dbl)  [unwired: 1 in, 1 out]
    n51 = shared-variable ".\\Lift.lvlib\\Verticle_Mech_Low"() -> (w141:dbl)  [unwired: 1 in, 1 out]
    n52 = shared-variable ".\\DriveStatus.lvlib\\Yaw Wind"(w115) -> ()  [unwired: 1 in, 1 out]
    n53 = shared-variable ".\\Lift.lvlib\\Verticle_Sensor_Hi"() -> (w139:dbl)  [unwired: 1 in, 1 out]
    n54 = shared-variable ".\\Lift.lvlib\\Verticle_Mech_Hi"() -> (w138:dbl)  [unwired: 1 in, 1 out]
    n55 = call <vilib>:"WPI_DigitalInputGetValue.vi"("DigitalInputDevRef"=w174) -> ("Value"=w169:bool)  [unwired: 8 in, 2 out]
    n56 = call <vilib>:"WPI_DigitalInputGetValue.vi"("DigitalInputDevRef"=w173) -> ("Value"=w168:bool)  [unwired: 8 in, 2 out]
    n57 = call <vilib>:"WPI_DigitalInputGetValue.vi"("DigitalInputDevRef"=w171) -> ("Value"=w166:bool)  [unwired: 8 in, 2 out]
    n58 = call <vilib>:"WPI_DigitalInputGetValue.vi"("DigitalInputDevRef"=w184) -> ("Value"=w146:bool)  [unwired: 8 in, 2 out]
    n59 = call <vilib>:"WPI_DigitalInputGetValue.vi"("DigitalInputDevRef"=w172) -> ("Value"=w167:bool)  [unwired: 8 in, 2 out]
    n60 = call <vilib>:"WPI_DigitalInputGetValue.vi"("DigitalInputDevRef"=w170) -> ("Value"=w165:bool)  [unwired: 8 in, 2 out]
    n61 = call-poly <vilib>:"CTRE_Phoenix_MotorController_Get_Enhanced.vi"("PhoenixMotorControlDevRef"=w182) -> ("Pulse Width Position"=w122:i32)  [unwired: 9 in, 5 out]
    "Raw Lift Elevation" <- w122
    n62 = call-poly <vilib>:"CTRE_Phoenix_MotorController_Get_Enhanced.vi"("PhoenixMotorControlDevRef"=w183) -> ("Pulse Width Position"=w60:i32)  [unwired: 9 in, 5 out]
    "Raw Lift Rotation" <- w60
    n63 = call <vilib>:"WPI_EncoderGet.vi"("EncoderDevRef"=w180) -> ("Distance"=w136:dbl, "Rate"=→"Left Encoder":dbl)  [unwired: 5 in, 4 out]
    n64 = call <vilib>:"WPI_EncoderGet.vi"("EncoderDevRef"=w181) -> ("Distance"=→"RightDriveEncoder" →"Right Encoder":dbl)  [unwired: 5 in, 5 out]
    n65 = Subtract(x=w123, y=w64) -> (x-y=w113:dbl)
    n66 = Divide(x=w67, y=w66) -> (x/y=w65:dbl)
    "IMU LIft Rate" <- w65
    "IMU Rate Lift" <- w65
    n67 = Select(t=WPI_RelayValue."Off", s=w90, f=WPI_RelayValue."Forward" ("RelayValue")) -> (s? t:f=w92:T28)
    n68 = call-poly <vilib>:"NT Write Value.vi"("Numeric"="ledMode", "Name"="/limelight/ledMode" ("ledmode")) -> ()  [unwired: 9 in, 1 out]
    n69 = call-poly <vilib>:"NT Write Value.vi"("Numeric"="pipeline", "Name"="/limelight/pipeline" ("pipeline")) -> ()  [unwired: 9 in, 1 out]
    n70 = call-poly <vilib>:"NT Write Value.vi"("Numeric"="userMode", "Name"="/limelight/camMode" ("pipeline")) -> ()  [unwired: 9 in, 1 out]
    n71 = call <vilib>:"WPI_RelaySet.vi"("RelayValue"=w92, "RelayDevRef"=w135) -> ()  [unwired: 8 in, 2 out]
    n72 = Not(x=w169) -> (.not. x?=w117:bool)
    "Cube? 3" <- w117
    n73 = Not(x=w168) -> (.not. x?=w118:bool)
    "Cube? 5" <- w118
    n74 = Not(x=w166) -> (.not. x?=w119:bool)
    "Cube? 1" <- w119
    n75 = Not(x=w146) -> (.not. x?=w134:bool)
    "Cube? 4" <- w134
    n76 = Not(x=w167) -> (.not. x?=w131:bool)
    "Cube? 6" <- w131
    n77 = Not(x=w165) -> (.not. x?=w133:bool)
    "Cube? 2" <- w133
    n78 = shared-variable ".\\LiftStatus.lvlib\\Lift Roll"(w129) -> ()  [unwired: 1 in, 1 out]
    n79 = Not(x="Reset Lift Rate") -> (.not. x?=w70:bool)
    n80 = shared-variable ".\\DriveStatus.lvlib\\Roll Wind"(w154) -> ()  [unwired: 1 in, 1 out]
    n81 = feedback #5(w65) -> (w75:dbl)
    n82 = Bundle By Name(cluster=cluster{"Sensor Low":dbl, "Sensor Hi":dbl} {"Sensor Low"=0.0, "Sensor Hi"=0.0} ("Sensor Config"), "Sensor Low"=w140, "Sensor Hi"=w139) -> (w157:cluster{"Sensor Low":dbl, "Sensor Hi":dbl})
    n83 = Max & Min(x=w65, y=w75) -> (max(x,y)=w72:dbl)  [unwired: 1 out]
    n84 = call <userlib>:"BoundAngle.vi"("Type"=T29."[-180, 180]", "Angle"=w113) -> ("Bound Angle"=w109:dbl)
    "Pitch LiftArm" <- w109
    n85 = Bundle By Name(cluster=cluster{"Mechanism Hi":dbl, "Mechanism Low":dbl} {"Mechanism Hi"=0.0, "Mechanism Low"=0.0} ("Mech Config"), "Mechanism Hi"=w149, "Mechanism Low"=w163) -> (w106:cluster{"Mechanism Hi":dbl, "Mechanism Low":dbl})
    n86 = Bundle By Name(cluster=cluster{"Mechanism Hi":dbl, "Mechanism Low":dbl} {"Mechanism Hi"=0.0, "Mechanism Low"=0.0} ("Mech Config"), "Mechanism Hi"=w138, "Mechanism Low"=w141) -> (w158:cluster{"Mechanism Hi":dbl, "Mechanism Low":dbl})
    n87 = Select(t=w72, s=w70, f=0.0) -> (s? t:f=w71:dbl)
    "IMU Lift Max Rate" <- w71
    n88 = feedback-in #5(w71) -> ()
    n89 = Bundle By Name(cluster=cluster{"Sensor Low":dbl, "Sensor Hi":dbl} {"Sensor Low"=0.0, "Sensor Hi"=0.0} ("Sensor Config"), "Sensor Low"=w148, "Sensor Hi"=w147) -> (w105:cluster{"Sensor Low":dbl, "Sensor Hi":dbl})
    n90 = shared-variable ".\\LiftStatus.lvlib\\Lift Pitch"(w109) -> ()  [unwired: 1 in, 1 out]
    n91 = shared-variable ".\\DriveStatus.lvlib\\Pitch Wind"(w153) -> ()  [unwired: 1 in, 1 out]
    n92 = Greater?(x=w109, y=120.0) -> (0:w110:bool)
    "Lift IMU Fault" <- w110
    n93 = call <userlib>:"LinearSensorCal.vi"("Sensor Config"=w157, "Mech Config"=w158, "Sense"=w122) -> ("Cal Sense"=→"LiftElevation":dbl)  [unwired: 8 in]
    n94 = call <userlib>:"LinearSensorCal.vi"("Sensor Config"=w105, "Mech Config"=w106, "Sense"=w60) -> ("Cal Sense"=w104:dbl)  [unwired: 8 in]
    "LiftRotation" <- w104
    n95 = shared-variable ".\\DevRefs.lvlib\\Drive DevRef Out"() -> (w85:T36)  [unwired: 1 in, 1 out]
    n96 = shared-variable ".\\LiftStatus.lvlib\\Lift IMU Failed?"(w110) -> ()  [unwired: 1 in, 1 out]
    n97 = Negate(x=w136) -> (-x=w152:dbl)
    "LeftDriveEncoder" <- w152
    n98 = shared-variable ".\\DevRefs.lvlib\\Drive DevRef Out"() -> (w114:T36)  [unwired: 1 in, 1 out]
    n99 = shared-variable ".\\LiftStatus.lvlib\\Verticle_Position"(w122) -> ()  [unwired: 1 in, 1 out]
    n100 = call-poly <vilib>:"NT Read Value.vi"("Name"="/limelight/tv") -> ("Numeric"=w99:dbl)  [unwired: 9 in, 1 out]
    n101 = call-poly <vilib>:"NT Read Value.vi"("Name"="/limelight/tx") -> ("Numeric"=w87:dbl)  [unwired: 9 in, 1 out]
    "tx" <- w87
    n102 = shared-variable ".\\Lift.lvlib\\Rotation_Mech_Low_Tuning"("Rotation_Mech_Low") -> ()  [unwired: 1 in, 1 out]
    n103 = shared-variable ".\\Lift.lvlib\\Rotation_Mech_Hi_Tuning"("Rotation_Mech_Hi") -> ()  [unwired: 1 in, 1 out]
    n104 = shared-variable ".\\Lift.lvlib\\Rotation_Sensor_Low_Tuning"("Rotation_Sensor_Low") -> ()  [unwired: 1 in, 1 out]
    n105 = shared-variable ".\\Lift.lvlib\\Rotation_Sensor_Hi_Tuning"("Rotation_Sensor_Hi") -> ()  [unwired: 1 in, 1 out]
    n106 = shared-variable ".\\Lift.lvlib\\Verticle_Mech_Hi_Tuning"("Verticle_Mech_Hi") -> ()  [unwired: 1 in, 1 out]
    n107 = shared-variable ".\\Lift.lvlib\\Verticle_Mech_Low_Tuning"("Verticle_Mech_Low") -> ()  [unwired: 1 in, 1 out]
    n108 = shared-variable ".\\Lift.lvlib\\Verticle_Sensor_Low_Tuning"("Verticle_Sensor_Low") -> ()  [unwired: 1 in, 1 out]
    n109 = shared-variable ".\\Lift.lvlib\\Verticle_Sensor_Hi_Tuning"("Verticle_Sensor_Hi") -> ()  [unwired: 1 in, 1 out]
    n110 = Select(t=w109, s="Lift Is IMU?", f=w104) -> (s? t:f=w108:dbl)
    n111 = Greater Than 0?(x=w99) -> (x > 0?=w86:bool)
    "Valid Target" <- w86
    n112 = Compound Arithmetic op=OR(w117, w118, w119, w134, w131, w133) -> (invert w132:bool)
    n113 = shared-variable ".\\DevRefs.lvlib\\Drive DevRef Out"() -> (w177:T36)  [unwired: 1 in, 1 out]
    n114 = shared-variable ".\\LiftStatus.lvlib\\Rotational_Position"(w108) -> ()  [unwired: 1 in, 1 out]
    n115 = shared-variable ".\\Camera.lvlib\\Horizontal_Offset"(w87) -> ()  [unwired: 1 in, 1 out]
    n116 = shared-variable ".\\Camera.lvlib\\Valid_Target?"(w86) -> ()  [unwired: 1 in, 1 out]
    n117 = call <userlib>:"Drive_Sensor_Yaw_Write.vi"("Angle"=w115, "Drive DevRef In"=w114) -> ()  [unwired: 10 in]
    n118 = call <userlib>:"JK_Latch.vi"("Reset"=w132, "Set"=FALSE) -> ("Q"=w116:bool)  [unwired: 5 in]
    n119 = Or(x="Cube? Fakeout", y=w116) -> (x .or. y?=w121:bool)
    "Cube?" <- w121
    n120 = call <userlib>:"Drive_Sensor_Camera_Write.vi"("Valid"=w86, "Angle"=w87, "Drive DevRef In"=w85) -> ()  [unwired: 9 in]
    n121 = shared-variable ".\\IntakeStatus.lvlib\\Cube?"(w121) -> ()  [unwired: 1 in, 1 out]
    n122 = call <userlib>:"Drive_Sensor_Distance_Write.vi"("Distance"=w152, "Drive DevRef In"=w177) -> ()  [unwired: 10 in]
    n123 = node-c288("SensorPeriod") -> ()  [unwired: 1 out]
  }
  n124 = node-c288(w30) -> ()  [unwired: 1 out]
  n125 = node-c288() -> (w33:T15)  [unwired: 4 in]
  n126 = node-c288() -> (w21:T15)  [unwired: 4 in]
  n127 = timed-loop {
    timing: w33 -> [_]
    timing-out: [_] -> w32
    stop <- _ stop-if-true
    n128 = node-c288() -> (→"QCP Finished Late? [i-1]":bool, →"QCP Iteration Duration":i64)  [unwired: 1 in]
    n129 = shared-variable ".\\DevRefs.lvlib\\Auto_QCP_DevRef"() -> (w209:T38)  [unwired: 1 in, 1 out]
    n130 = shared-variable ".\\DevRefs.lvlib\\Lift_QCP_DevRef"() -> (w211:T38)  [unwired: 1 in, 1 out]
    n131 = shared-variable ".\\DevRefs.lvlib\\Sensor_QCP_DevRef_Out"() -> (w208:T38)  [unwired: 1 in, 1 out]
    n132 = shared-variable ".\\DevRefs.lvlib\\Drive_QCP_DevRef"() -> (w210:T38)  [unwired: 1 in, 1 out]
    n133 = shared-variable ".\\DevRefs.lvlib\\Intake_QCP_DevRef"() -> (w212:T38)  [unwired: 1 in, 1 out]
    n134 = call <userlib>:"Signal_Pulse.vi"("Input"="SensorWriteQCPFile") -> ("Output"=w241:bool)
    n135 = call <userlib>:"Signal_Pulse.vi"("Input"="LiftWriteQCPFile") -> ("Output"=w243:bool)
    n136 = call <userlib>:"Signal_Pulse.vi"("Input"="DriveWriteQCPFile") -> ("Output"=w249:bool)
    n137 = call <userlib>:"Signal_Pulse.vi"("Input"="AutoWriteQCPFile") -> ("Output"=w247:bool)
    n138 = call <userlib>:"Signal_Pulse.vi"("Input"="IntakeWriteQCPFile") -> ("Output"=w245:bool)
    n139 = case shown="True" w247 {
      tunnel: w209 -> [_ w307]
      frame False {
      }
      frame True {
        n140 = call <userlib>:"QCP_WriteFile.vi"("Overrite?"=TRUE, "Path"="/home/lvuser/QCP_Files/AutoConfig.qcp", "QCP_DevRef_In"=w307) -> ()  [unwired: 7 in, 2 out]
      }
    }
    n141 = case shown="True" w241 {
      tunnel: w208 -> [_ w298]
      frame False {
      }
      frame True {
        n142 = call <userlib>:"QCP_WriteFile.vi"("Overrite?"=TRUE, "Path"="/home/lvuser/QCP_Files/Sensor_Loop.qcp", "QCP_DevRef_In"=w298) -> ()  [unwired: 7 in, 2 out]
      }
    }
    n143 = case shown="True" w249 {
      tunnel: w210 -> [_ w310]
      frame False {
      }
      frame True {
        n144 = call <userlib>:"QCP_WriteFile.vi"("Overrite?"=TRUE, "Path"="/home/lvuser/QCP_Files/Drive.qcp", "QCP_DevRef_In"=w310) -> ()  [unwired: 7 in, 2 out]
      }
    }
    n145 = case shown="True" w245 {
      tunnel: w212 -> [_ w304]
      frame False {
      }
      frame True {
        n146 = call <userlib>:"QCP_WriteFile.vi"("Overrite?"=TRUE, "Path"="/home/lvuser/QCP_Files/Intake.qcp", "QCP_DevRef_In"=w304) -> ()  [unwired: 7 in, 2 out]
      }
    }
    n147 = case shown="True" w243 {
      tunnel: w211 -> [_ w301]
      frame False {
      }
      frame True {
        n148 = call <userlib>:"QCP_WriteFile.vi"("Overrite?"=TRUE, "Path"="/home/lvuser/QCP_Files/Lift.qcp", "QCP_DevRef_In"=w301) -> ()  [unwired: 7 in, 2 out]
      }
    }
    n149 = First Call?() -> (First Call?: T/F=w191:bool)
    n150 = feedback #6() -> (w239:bool)  [unwired: 1 in]
    n151 = feedback-in #6("LiftTuningMode?") -> ()
    n152 = feedback #7() -> (w238:bool)  [unwired: 1 in]
    n153 = feedback-in #7("DriveTuningMode?") -> ()
    n154 = feedback #8() -> (w232:bool)  [unwired: 1 in]
    n155 = feedback-in #8("SensorTuningMode?") -> ()
    n156 = feedback #9() -> (w236:bool)  [unwired: 1 in]
    n157 = feedback-in #9("AutoTuningMode?") -> ()
    n158 = feedback #10() -> (w234:bool)  [unwired: 1 in]
    n159 = feedback-in #10("IntakeTuningMode?") -> ()
    n160 = Not Equal?(x="LiftTuningMode?", y=w239) -> (x != y?=w202:bool)
    n161 = Not Equal?(x="DriveTuningMode?", y=w238) -> (x != y?=w237:bool)
    n162 = Not Equal?(x="SensorTuningMode?", y=w232) -> (x != y?=w231:bool)
    n163 = Not Equal?(x="AutoTuningMode?", y=w236) -> (x != y?=w235:bool)
    n164 = Not Equal?(x="IntakeTuningMode?", y=w234) -> (x != y?=w233:bool)
    n165 = And(x="LiftTuningMode?", y=w191) -> (x .and. y?=w201:bool)
    n166 = And(x="DriveTuningMode?", y=w191) -> (x .and. y?=w199:bool)
    n167 = And(x="AutoTuningMode?", y=w191) -> (x .and. y?=w192:bool)
    n168 = And(x="IntakeTuningMode?", y=w191) -> (x .and. y?=w196:bool)
    n169 = And(x="SensorTuningMode?", y=w191) -> (x .and. y?=w194:bool)
    n170 = Or(x=w202, y=w201) -> (x .or. y?=w203:bool)
    n171 = Or(x=w235, y=w192) -> (x .or. y?=w205:bool)
    n172 = Or(x=w237, y=w199) -> (x .or. y?=w204:bool)
    n173 = Or(x=w231, y=w194) -> (x .or. y?=w207:bool)
    n174 = Or(x=w233, y=w196) -> (x .or. y?=w206:bool)
    n175 = shared-variable ".\\LiftStatus.lvlib\\LiftTuningMode"("LiftTuningMode?") -> ()  [unwired: 1 in, 1 out]
    n176 = case shown="True" w203 {
      tunnel: "LiftTuningMode?" -> [_ w296]
      tunnel: w211 -> [_ w295]
      frame False {
      }
      frame True {
        n177 = call <userlib>:"QCP_TuningModeSet.vi"("On?"=w296, "QCP_DevRef_In"=w295) -> ()  [unwired: 8 in, 2 out]
      }
    }
    n178 = case shown="True" w204 {
      tunnel: "DriveTuningMode?" -> [_ w294]
      tunnel: w210 -> [_ w293]
      frame False {
      }
      frame True {
        n179 = call <userlib>:"QCP_TuningModeSet.vi"("On?"=w294, "QCP_DevRef_In"=w293) -> ()  [unwired: 8 in, 2 out]
      }
    }
    n180 = case shown="True" w207 {
      tunnel: "SensorTuningMode?" -> [_ w288]
      tunnel: w208 -> [_ w287]
      frame False {
      }
      frame True {
        n181 = call <userlib>:"QCP_TuningModeSet.vi"("On?"=w288, "QCP_DevRef_In"=w287) -> ()  [unwired: 8 in, 2 out]
      }
    }
    n182 = case shown="True" w205 {
      tunnel: "AutoTuningMode?" -> [_ w292]
      tunnel: w209 -> [_ w291]
      frame False {
      }
      frame True {
        n183 = call <userlib>:"QCP_TuningModeSet.vi"("On?"=w292, "QCP_DevRef_In"=w291) -> ()  [unwired: 8 in, 2 out]
      }
    }
    n184 = case shown="True" w206 {
      tunnel: "IntakeTuningMode?" -> [_ w290]
      tunnel: w212 -> [_ w289]
      frame False {
      }
      frame True {
        n185 = call <userlib>:"QCP_TuningModeSet.vi"("On?"=w290, "QCP_DevRef_In"=w289) -> ()  [unwired: 8 in, 2 out]
      }
    }
    n186 = call <userlib>:"Signal_Pulse.vi"("Input"="Read Sensor QCP") -> ("Output"=w225:bool)
    n187 = call <userlib>:"Signal_Pulse.vi"("Input"="Read Auto QCP") -> ("Output"=w227:bool)
    n188 = call <userlib>:"Signal_Pulse.vi"("Input"="Read Drive QCP") -> ("Output"=w228:bool)
    n189 = call <userlib>:"Signal_Pulse.vi"("Input"="Read Intake QCP") -> ("Output"=w226:bool)
    n190 = call <userlib>:"Signal_Pulse.vi"("Input"="Read Lift QCP") -> ("Output"=w229:bool)
    n191 = case shown="True" w225 {
      tunnel: w208 -> [_ w259]
      tunnel: [FALSE ("Overrite Existing Data?") w255] -> w217
      frame False {
      }
      frame True {
        w255 = TRUE ("Overrite Existing Data?")
        n192 = call <userlib>:"QCP_ReadFile.vi"("Overrite Existing Data?"=w255, "Same Name Fail?"=FALSE, "Path Relative?"=FALSE, "Path"="/home/lvuser/QCP_Files/Sensor_Loop.qcp", "QCP_DevRef_In"=w259) -> ("QCP_DevRef_Out"=w254:T39)  [unwired: 5 in, 1 out]
        n193 = shared-variable ".\\DevRefs.lvlib\\Sensor_QCP_DevRef_Out"(w254) -> ()  [unwired: 1 in, 1 out]
      }
    }
    n194 = case shown="True" w227 {
      tunnel: w209 -> [_ w272]
      frame False {
      }
      frame True {
        n195 = call <userlib>:"QCP_ReadFile.vi"("Overrite Existing Data?"=TRUE, "Same Name Fail?"=FALSE, "Path Relative?"=FALSE, "Path"="/home/lvuser/QCP_Files/AutoConfig.qcp", "QCP_DevRef_In"=w272) -> ("QCP_DevRef_Out"=w267:T39)  [unwired: 5 in, 1 out]
        n196 = shared-variable ".\\DevRefs.lvlib\\Auto_QCP_DevRef"(w267) -> ()  [unwired: 1 in, 1 out]
      }
    }
    n197 = case shown="True" w226 {
      tunnel: w212 -> [_ w266]
      tunnel: [FALSE ("Overrite Existing Data?") w262] -> w219
      frame False {
      }
      frame True {
        w262 = TRUE ("Overrite Existing Data?")
        n198 = call <userlib>:"QCP_ReadFile.vi"("Overrite Existing Data?"=w262, "Same Name Fail?"=FALSE, "Path Relative?"=FALSE, "Path"="/home/lvuser/QCP_Files/Intake.qcp", "QCP_DevRef_In"=w266) -> ("QCP_DevRef_Out"=w261:T39)  [unwired: 5 in, 1 out]
        n199 = shared-variable ".\\DevRefs.lvlib\\Intake_QCP_DevRef"(w261) -> ()  [unwired: 1 in, 1 out]
      }
    }
    n200 = case shown="True" w229 {
      tunnel: w211 -> [_ w286]
      tunnel: [FALSE ("Overrite Existing Data?") w282] -> w213
      frame False {
      }
      frame True {
        w282 = TRUE ("Overrite Existing Data?")
        n201 = call <userlib>:"QCP_ReadFile.vi"("Overrite Existing Data?"=w282, "Same Name Fail?"=FALSE, "Path Relative?"=FALSE, "Path"="/home/lvuser/QCP_Files/Lift.qcp", "QCP_DevRef_In"=w286) -> ("QCP_DevRef_Out"=w281:T39)  [unwired: 5 in, 1 out]
        n202 = shared-variable ".\\DevRefs.lvlib\\Lift_QCP_DevRef"(w281) -> ()  [unwired: 1 in, 1 out]
      }
    }
    n203 = case shown="True" w228 {
      tunnel: w210 -> [_ w279]
      tunnel: [FALSE ("Overrite Existing Data?") w275] -> w215
      frame False {
      }
      frame True {
        w275 = TRUE ("Overrite Existing Data?")
        n204 = call <userlib>:"QCP_ReadFile.vi"("Overrite Existing Data?"=w275, "Same Name Fail?"=FALSE, "Path Relative?"=FALSE, "Path"="/home/lvuser/QCP_Files/Drive.qcp", "QCP_DevRef_In"=w279) -> ("QCP_DevRef_Out"=w274:T39)  [unwired: 5 in, 1 out]
        n205 = shared-variable ".\\DevRefs.lvlib\\Drive_QCP_DevRef"(w274) -> ()  [unwired: 1 in, 1 out]
      }
    }
    n206 = Compound Arithmetic op=OR(w213, "LiftTuningMode?", w191) -> (w214:bool)
    n207 = Compound Arithmetic op=OR(w215, "DriveTuningMode?", w191) -> (w216:bool)
    n208 = Compound Arithmetic op=OR(w219, "IntakeTuningMode?", w191) -> (w220:bool)
    n209 = Compound Arithmetic op=OR(w217, "SensorTuningMode?", w191) -> (w218:bool)
    n210 = case shown="True" w214 {
      frame False {
      }
      frame True {
        n211 = call "Lift.vi"() -> ()  [unwired: 12 in]
      }
    }
    n212 = case shown="True" w216 {
      frame False {
      }
      frame True {
        n213 = call "DriveLoop.vi"() -> ()  [unwired: 12 in]
      }
    }
    n214 = case shown="True" w220 {
      frame False {
      }
      frame True {
        n215 = call "Intake.vi"() -> ()  [unwired: 12 in]
      }
    }
    n216 = case shown="True" w218 {
      frame False {
      }
      frame True {
        n217 = call "SensorLoop.vi"() -> ()  [unwired: 12 in]
      }
    }
    n218 = node-c288("QCPPeriod") -> ()  [unwired: 1 out]
  }
  n219 = timed-loop {
    timing: w21 -> [_]
    timing-out: [_] -> w20
    stop <- _ stop-if-true
    n220 = node-c288() -> (→"PID Finished Late? [i-1]":bool, →"PID Iteration Duration":i64)  [unwired: 1 in]
    n221 = First Call?() -> (First Call?: T/F=w318:bool)
    n222 = call <userlib>:"Signal_Pulse.vi"("Input"="Update PID") -> ("Output"=w319:bool)
    n223 = Or(x=w318, y=w319) -> (x .or. y?=w320:bool)
    n224 = case shown="True" w320 {
      frame False {
      }
      frame True {
        n225 = shared-variable ".\\DevRefs.lvlib\\Drive DevRef Out"() -> (w325:T36)  [unwired: 1 in, 1 out]
        n226 = Bundle By Name(cluster=T6 {"Yaw, Driving Straight"={"proportional gain (Kc)"=1.0, "integral time (Ti, min)"=0.01, "derivative time (Td, min)"=0.0}, "Yaw, Holding Still"={"proportional gain (Kc)"=1.0, "integral time (Ti, min)"=0.01, "derivative time (Td, min)"=0.0}, "Distance, Driving Straight"={"proportional gain (Kc)"=1.0, "integral time (Ti, min)"=0.01, "derivative time (Td, min)"=0.0}, "Distance, Holding Still"={"proportional gain (Kc)"=1.0, "integral time (Ti, min)"=0.01, "derivative time (Td, min)"=0.0}} ("PID Gains"), "Yaw, Driving Straight"="Yaw_Driving_Straight_PID_gains", "Yaw, Holding Still"="Yaw_Holding_Still_PID_Gains", "Distance, Driving Straight"="Distance_Driving_Straight_PID_Gains", "Distance, Holding Still"="Distance_Holding_Still_PID_gains") -> (w330:T6)
        n227 = call-poly <userlib>:"Drive_Loop_Command.vi"("PID Gains"=w330, "Control Cluster"=w325) -> ()  [unwired: 10 in]
      }
    }
    n228 = node-c288("PIDPeriod") -> ()  [unwired: 1 out]
  }
  n229 = node-c288(w20) -> ()  [unwired: 1 out]
  n230 = call <vilib>:"WPI_ServoRefNum Registry Get.vi"("refnum name"="LiftBrake") -> ("ServoDeviceRef"=w2:T40)  [unwired: 9 in, 1 out]
  n231 = while {
    tunnel: w2 -> [w341]
    stop <- FALSE stop-if-true
    n232 = call <vilib>:"WPI_ServoSetPosition.vi"("Position"="Position", "ServoDeviceRef"=w341) -> ()  [unwired: 8 in, 2 out]
    n233 = Wait (ms)(milliseconds to wait=u32 300) -> ()  [unwired: 1 out]
  }
  n234 = node-c288(w32) -> ()  [unwired: 1 out]
  n235 = node-c288() -> (w19:T15)  [unwired: 4 in]
  n236 = Bundle By Name(cluster=T6 {"Yaw, Driving Straight"={"proportional gain (Kc)"=1.0, "integral time (Ti, min)"=0.01, "derivative time (Td, min)"=0.0}, "Yaw, Holding Still"={"proportional gain (Kc)"=1.0, "integral time (Ti, min)"=0.01, "derivative time (Td, min)"=0.0}, "Distance, Driving Straight"={"proportional gain (Kc)"=1.0, "integral time (Ti, min)"=0.01, "derivative time (Td, min)"=0.0}, "Distance, Holding Still"={"proportional gain (Kc)"=1.0, "integral time (Ti, min)"=0.01, "derivative time (Td, min)"=0.0}} ("Init PID Gains"), "Yaw, Driving Straight"=w5, "Yaw, Holding Still"=w5, "Distance, Driving Straight"=w4, "Distance, Holding Still"=w4) -> (w3:T6)
  n237 = shared-variable ".\\DevRefs.lvlib\\Drive DevRef Out"() -> (w17:T36)  [unwired: 1 in, 1 out]
  n238 = timed-loop {
    timing: w19 -> [_]
    timing-out: [_] -> w18
    tunnel: w17 -> [w349]
    shift-right: [w350] -> _
    shift-left: DriveCommands."Manual" -> [w351]
    stop <- _ stop-if-true
    n239 = node-c288() -> (→"DriveFinished Late? [i-1]":bool, →"Drive Iteration Duration":i64)  [unwired: 1 in]
    n240 = shared-variable ".\\DevRefs.lvlib\\DriveNotifier"() -> (w354:refnum<notifier>)  [unwired: 1 in, 1 out]
    n241 = Wait on Notification(notifier=w354, timeout in ms (-1)=0) -> (notification=w352:T5, timed out?=w353:bool)  [unwired: 2 in, 2 out]
    n242 = case shown="True" w353 {
      tunnel: w349 -> [w360 w374]
      tunnel: w352 -> [w359 _]
      tunnel: w351 -> [_ w373]
      tunnel: [w359 w373] -> w350
      frame False {
        n243 = case shown="\"Acquire Cube\"" w359 {
          tunnel: w360 -> [_ w363 _ w368]
          frame "Manual", Default {
          }
          frame "Acquire Cube" {
            n244 = shared-variable ".\\DriveLoop.lvlib\\Acquire_Cube_Speed"() -> (w362:dbl)  [unwired: 1 in, 1 out]
            n245 = shared-variable ".\\Joystick.lvlib\\Axis_1"() -> (w361:dbl)  [unwired: 1 in, 1 out]
            n246 = shared-variable ".\\DriveLoop.lvlib\\Acquire_Cube_Speed_Tuning"("AquireSpeed") -> ()  [unwired: 1 in, 1 out]
            n247 = call-poly <userlib>:"Drive_Loop_Command.vi"("Forward Power"=w361, "Max Turn Power"=w362, "Drive Loop Cluster"=w363) -> ()  [unwired: 8 in, 1 out]
          }
          frame "Drive Path" {
          }
          frame "Center on Cube" {
            n248 = shared-variable ".\\DriveLoop.lvlib\\Center_On_Cube_Tolerance"() -> (w366:dbl)  [unwired: 1 in, 1 out]
            n249 = shared-variable ".\\DriveLoop.lvlib\\Center_On_Cube_Tolerance_Tuning"("CenterOnCubeTolerance") -> ()  [unwired: 1 in, 1 out]
            n250 = Negate(x=w366) -> (-x=w371:dbl)
            n251 = Bundle By Name(cluster=T41 {"Distance"={"Upper Error Bound"=0.0, "Lower Error Bound"=0.0}, "Yaw"={"Upper Error Bound"=0.0, "Lower Error Bound"=0.0}} ("Tolerance Settings"), "Yaw.Upper Error Bound"=w366, "Yaw.Lower Error Bound"=w371) -> (w372:T41)
            n252 = shared-variable ".\\DriveLoop.lvlib\\Center_Speed"() -> (w369:dbl)  [unwired: 1 in, 1 out]
            n253 = shared-variable ".\\DriveLoop.lvlib\\Center_Speed_Tuning"("CenterSpeed") -> ()  [unwired: 1 in, 1 out]
            n254 = call <userlib>:"Drive_Update_Tolerance.vi"("Tolerance Settings"=w372, "Drive DevRef In"=w368) -> ()  [unwired: 10 in]
            n255 = call-poly <userlib>:"Drive_Loop_Command.vi"("Max Turn Power"=w369, "Drive Loop Cluster"=w368) -> ()  [unwired: 9 in, 1 out]
          }
        }
      }
      frame True {
        n256 = case shown="\"Manual\", Default" w373 {
          tunnel: w374 -> [w435 w441 w446 _]
          frame "Manual", Default {
            n257 = shared-variable ".\\LiftStatus.lvlib\\Lift_Command"() -> (w409:T2)  [unwired: 1 in, 1 out]
            n258 = shared-variable ".\\Joystick.lvlib\\Axis_2"() -> (w401:dbl)  [unwired: 1 in, 1 out]
            n259 = Equal?(x=w409, y=T2."To Scale Low") -> (x = y?=w405:bool)
            n260 = Equal?(x=w409, y=T2."To Scale Medium") -> (x = y?=w404:bool)
            n261 = Equal?(x=w409, y=T2."To Scale High") -> (x = y?=w403:bool)
            n262 = Square(x=w401) -> (x^2=w399:dbl)
            n263 = Sign(1:w401) -> (0:w400:dbl)
            n264 = Multiply(x=w400, y=w399) -> (x*y=w402:dbl)
            n265 = shared-variable ".\\Joystick.lvlib\\Axis_1"() -> (w428:dbl)  [unwired: 1 in, 1 out]
            n266 = Select(t=w402, s="Square Wheel", f=w401) -> (s? t:f=w426:dbl)
            n267 = Multiply(x="Steer Scale", y=w426) -> (x*y=w422:dbl)
            n268 = Square(x=w428) -> (x^2=w433:dbl)
            n269 = call <userlib>:"Deadzone.vi"("Deadzone"="Turn In Place Deadband", "Input Signal"=w428) -> ("In Deadzone?"=w427:bool)  [unwired: 1 out]
            n270 = shared-variable ".\\Voltage Reg.lvlib\\Above threshold voltage?"() -> (w375:bool)  [unwired: 1 in, 1 out]
            n271 = Sign(1:w428) -> (0:w432:dbl)
            n272 = shared-variable ".\\DriveStatus.lvlib\\Slow Mode?"() -> (w410:bool)  [unwired: 1 in, 1 out]
            n273 = Multiply(x=w432, y=w433) -> (x*y=w431:dbl)
            n274 = Select(t=w401, s=w427, f=w422) -> (s? t:f=w419:dbl)
            n275 = Select(t=w431, s="Square Throttle", f=w428) -> (s? t:f=w425:dbl)
            n276 = And(x=w375, y="Current Limit?") -> (x .and. y?=w378:bool)
            n277 = Multiply(x=w425, y="Throttle Scale") -> (x*y=w421:dbl)
            n278 = Compound Arithmetic op=OR(w378, w410, w405, w404, w403) -> (w411:bool)
            n279 = Select(t="Throttle Slow Mode Mult", s=w411, f=1.0) -> (s? t:f=w416:dbl)
            n280 = Select(t="Steer Slow Mode Mult", s=w411, f=1.0) -> (s? t:f=w413:dbl)
            n281 = feedback #11() -> (w389:dbl)  [unwired: 1 in]
            n282 = feedback #12() -> (w388:dbl)  [unwired: 1 in]
            n283 = Absolute Value(x=w389) -> (abs(x)=w393:dbl)
            n284 = feedback #13() -> (w391:dbl)  [unwired: 1 in]
            n285 = feedback-in #13(w389) -> ()
            n286 = feedback-in #14(w388) -> ()
            n287 = feedback #14() -> (w390:dbl)  [unwired: 1 in]
            n288 = Absolute Value(x=w391) -> (abs(x)=w392:dbl)
            n289 = Absolute Value(x=w388) -> (abs(x)=w394:dbl)
            n290 = Absolute Value(x=w390) -> (abs(x)=w395:dbl)
            n291 = Greater?(x=w393, y=w392) -> (0:w380:bool)
            n292 = Greater?(x=w394, y=w395) -> (0:w383:bool)
            n293 = Select(t="Acceleration Steer Rate Limit", s=w383, f="Deceleration Steer Rate Limit") -> (s? t:f=w385:dbl)
            n294 = Multiply(x=w421, y=w416) -> (x*y=w420:dbl)
            n295 = Multiply(x=w419, y=w413) -> (x*y=w418:dbl)
            n296 = Select(t="Acceleration Throttle Rate Limit", s=w380, f="DecelerationThrottle Rate Limit") -> (s? t:f=w381:dbl)
            n297 = call <vilib>:"WPI_DriverStationGetModeAndStatus.vi"() -> ("Robot Mode"=w398:T43)  [unwired: 10 in, 1 out]
            n298 = call-poly <vilib>:"PID Output Rate Limiter.vi"("output rate (EGU/min)"=w381, "initial output"=w420, "input (controller output)"=w420) -> ("output"=w387:dbl)  [unwired: 5 in, 1 out]
            n299 = feedback-in #11(w387) -> ()
            n300 = call-poly <vilib>:"PID Output Rate Limiter.vi"("output rate (EGU/min)"=w385, "initial output"=w418, "input (controller output)"=w418) -> ("output"=w376:dbl)  [unwired: 5 in, 1 out]
            "Steer Fed Value" <- w376
            n301 = feedback-in #12(w376) -> ()
            n302 = Not Equal?(x=w398, y=WPI_DriverStationRobotMode2."Autonomous Enabled") -> (x != y?=w396:bool)
            n303 = case shown="True" w396 {
              tunnel: w435 -> [_ w438]
              tunnel: w387 -> [_ w437]
              tunnel: w376 -> [_ w436]
              frame False {
              }
              frame True {
                n304 = call-poly <userlib>:"Drive_Loop_Command.vi"("Wheel"=w436, "Throttle"=w437, "Drive Loop Cluster"=w438) -> ()  [unwired: 8 in, 1 out]
              }
            }
          }
          frame "Center on Cube" {
            n305 = call <userlib>:"GetCommandFinished.vi"("Type"=CmdFinishedTypes."Poll", "DriveDevRefIn"=w441) -> ("Finished?"=w439:bool)  [unwired: 8 in, 1 out]
            n306 = case shown="True" w439 {
              frame False {
              }
              frame True {
                n307 = shared-variable ".\\DevRefs.lvlib\\DriveNotifier"() -> (w443:refnum<notifier>)  [unwired: 1 in, 1 out]
                n308 = Send Notification(notification=DriveCommands."Acquire Cube" ("Enum"), notifier=w443) -> ()  [unwired: 1 in, 2 out]
              }
            }
          }
          frame "Acquire Cube" {
            n309 = shared-variable ".\\DriveLoop.lvlib\\Acquire_Cube_Speed"() -> (w445:dbl)  [unwired: 1 in, 1 out]
            n310 = shared-variable ".\\Joystick.lvlib\\Axis_1"() -> (w444:dbl)  [unwired: 1 in, 1 out]
            n311 = shared-variable ".\\IntakeStatus.lvlib\\Cube?"() -> (w447:bool)  [unwired: 1 in, 1 out]
            n312 = case shown="True" w447 {
              frame False {
              }
              frame True {
                n313 = shared-variable ".\\DevRefs.lvlib\\DriveNotifier"() -> (w449:refnum<notifier>)  [unwired: 1 in, 1 out]
                n314 = Send Notification(notification=DriveCommands."Manual" ("Enum"), notifier=w449) -> ()  [unwired: 1 in, 2 out]
              }
            }
            n315 = call-poly <userlib>:"Drive_Loop_Command.vi"("Forward Power"=w444, "Max Turn Power"=w445, "Drive Loop Cluster"=w446) -> ()  [unwired: 8 in, 1 out]
          }
          frame "Drive Path" {
          }
        }
      }
    }
    n316 = call <userlib>:"Drive_Loop_Get_PID_Inputs.vi"("Drive DevRef In"=w349) -> ("PID Values"=w345:T45)  [unwired: 10 in]
    n317 = Unbundle By Name(w345) -> ("EncoderPID.Setpoint"=w348:dbl, "EncoderPID.Process"=w347:dbl)
    n318 = Bundle("Setpoint"=w348, "Process"=w347) -> (→"Dist Resp":cluster{"Setpoint":dbl, "Process":dbl})  [unwired: 1 in]
    n319 = Unbundle By Name(w345) -> ("YawPID.Setpoint"=w344:dbl, "YawPID.Process"=w343:dbl)
    n320 = Bundle("Setpoint"=w344, "Process"=w343) -> (→"Angle Resp":cluster{"Setpoint":dbl, "Process":dbl})  [unwired: 1 in]
    n321 = node-c288("Drive Period") -> ()  [unwired: 1 out]
    "Drive Command" <- w351
  }
  n322 = call <userlib>:"Drive_Loop_Control_Loop.vi"("Init PID Gains"=w3, "Init Period"=i64 40, "Drive DevRef In"=w17) -> ()  [unwired: 9 in]
  n323 = node-c288(w18) -> ()  [unwired: 1 out]
  n324 = call <vilib>:"WPI_MotorControlRefNum Registry Get.vi"("refnum name"="Intake") -> ("MotorControlDevRef"=w14:T9)  [unwired: 9 in, 1 out]
  n325 = call <vilib>:"CTRE_Phoenix_MotorControl_RefNumRegistryGet.vi"("refnum name"="LiftElevation") -> ("PhoenixMotorControlDevRef"=w9:T9)  [unwired: 9 in, 1 out]
  n326 = call <vilib>:"WPI_ServoRefNum Registry Get.vi"("refnum name"="LiftBrake") -> ("ServoDeviceRef"=w7:T40)  [unwired: 9 in, 1 out]
  n327 = call <vilib>:"CTRE_Phoenix_MotorControl_RefNumRegistryGet.vi"("refnum name"="LiftRotation") -> ("PhoenixMotorControlDevRef"=w12:T9)  [unwired: 9 in, 1 out]
  n328 = disable-structure shown="Disabled" {
    frame Disabled {
      n329 = while {
        stop <- FALSE stop-if-true
        n330 = call-poly <vilib>:"WPI_Power Get Rail Voltage and Current.vi"() -> ("5 volt rail voltage (V)"=w468:dbl, "5 volt rail current (A)"=w467:dbl)  [unwired: 13 in, 1 out]
        "5 volt rail voltage (V)" <- w468
        "5 volt rail current (A)" <- w467
        n331 = call <vilib>:"WPI_Power Get roboRIO Rail Faults.vi"() -> ("Input Voltage Brown Out"=w466:bool, "3.3V User Rail Short"=w464:bool, "5 V User Rail Short"=w462:bool, "6 V User Rail Short"=w460:bool, "5V User Rail Brown Out"=w458:bool)  [unwired: 10 in, 1 out]
        n332 = call <userlib>:"Latch.vi"("In"=w458) -> ("Out"=→"5V User Rail Brown Out":bool)  [unwired: 1 in]
        n333 = call <userlib>:"Latch.vi"("In"=w462) -> ("Out"=→"5 V User Rail Short":bool)  [unwired: 1 in]
        n334 = call <userlib>:"Latch.vi"("In"=w460) -> ("Out"=→"6 V User Rail Short":bool)  [unwired: 1 in]
        n335 = call <userlib>:"Latch.vi"("In"=w466) -> ("Out"=→"Input Voltage Brown Out":bool)  [unwired: 1 in]
        n336 = call <userlib>:"Latch.vi"("In"=w464) -> ("Out"=→"3.3V User Rail Short":bool)  [unwired: 1 in]
        n337 = feedback #15(inf) -> (w477:dbl)
        n338 = Select(t=0.0, s="Reset Voltage Max", f=w477) -> (s? t:f=w476:dbl)
        n339 = Max & Min(x=w468, y=w476) -> (min(x,y)=w456:dbl)  [unwired: 1 out]
        "Voltage Min" <- w456
        n340 = feedback-in #15(w456) -> ()
        n341 = feedback #16(-inf) -> (w472:dbl)
        n342 = Select(t=0.0, s="Reset Current Max", f=w472) -> (s? t:f=w473:dbl)
        n343 = Max & Min(x=w467, y=w473) -> (max(x,y)=w469:dbl)  [unwired: 1 out]
        "5V Rail Current Max" <- w469
        n344 = feedback-in #16(w469) -> ()
        n345 = Wait (ms)(milliseconds to wait=u32 500) -> ()  [unwired: 1 out]
      }
    }
    frame Enabled {
    }
  }
  n346 = call "LV2Lift.vi"("VerticleMotorControlDevRef"=w9, "Brake DevRef"=w7, "RotationMotorControlDevRef"=w12) -> ()  [unwired: 13 in]
  n347 = call "Intake level 2.vi"("MotorControlDevRef"=w14) -> ()  [unwired: 10 in]
  n348 = while {
    stop <- FALSE stop-if-true
    n349 = shared-variable ".\\IntakeStatus.lvlib\\Intake Iteration Duration"() -> (→"Intake Iteration Duration":i64)  [unwired: 1 in, 1 out]
    n350 = shared-variable ".\\IntakeStatus.lvlib\\Intake Finished Late? [i-1]"() -> (→"Intake Finished Late? [i-1]":bool)  [unwired: 1 in, 1 out]
    n351 = shared-variable ".\\IntakeStatus.lvlib\\intake power out"() -> (→"Intake_Command":u16)  [unwired: 1 in, 1 out]
    n352 = shared-variable ".\\Intake.lvlib\\Intake_Motor_Power_Tuning"("Intake Speed") -> ()  [unwired: 1 in, 1 out]
    n353 = shared-variable ".\\IntakeStatus.lvlib\\Intake Period"("Intake Period") -> ()  [unwired: 1 in, 1 out]
    n354 = Wait (ms)(milliseconds to wait=u32 1000) -> ()  [unwired: 1 out]
  }
  n355 = while {
    stop <- FALSE stop-if-true
    n356 = shared-variable ".\\LiftStatus.lvlib\\Lift Iteration Duration"() -> (→"Lift Iteration Duration":i64)  [unwired: 1 in, 1 out]
    n357 = shared-variable ".\\LiftStatus.lvlib\\Lift Finished Late? [i-1]"() -> (→"Lift Finished Late? [i-1]":bool)  [unwired: 1 in, 1 out]
    n358 = shared-variable ".\\LiftStatus.lvlib\\Lift_Command"() -> (→"Lift_Command":T2)  [unwired: 1 in, 1 out]
    n359 = shared-variable ".\\LiftStatus.lvlib\\Lift Period"("Lift Period") -> ()  [unwired: 1 in, 1 out]
    n360 = Wait (ms)(milliseconds to wait=u32 1000) -> ()  [unwired: 1 out]
  }
  n361 = while {
    stop <- FALSE stop-if-true
    n362 = Wait (ms)(milliseconds to wait=u32 250) -> ()  [unwired: 1 out]
    n363 = feedback-in #17("PDP Channel") -> ()
    n364 = feedback #17() -> (w508:dbl)  [unwired: 1 in]
    n365 = call <vilib>:"WPI_Power Get PDP Currents.vi"("Power Distribution Panel (0)"=u8 50, "PDP Channel"="PDP Channel") -> ("current (A)"=w498:dbl, "all currents (A)"=w517:dbl[])  [unwired: 11 in, 1 out]
    "PDP Channel Current (A)" <- w498
    "Current (A)" <- w498
    n366 = Not Equal?(x="PDP Channel", y=w508) -> (x != y?=w507:bool)
    n367 = Add Array Elements(numeric array=w517) -> (sum=w497:dbl)
    "PDP Total Current" <- w497
    "Total Current (A)" <- w497
    n368 = call <userlib>:"Signal_Pulse.vi"("Input"="Reset Max Current?") -> ("Output"=w505:bool)
    n369 = call <userlib>:"Signal_Pulse.vi"("Input"=w507) -> ("Output"=w501:bool)
    n370 = call <userlib>:"Signal_Pulse.vi"("Input"="Reet Max Total") -> ("Output"=w502:bool)
    n371 = Or(x=w505, y=w501) -> (x .or. y?=w504:bool)
    n372 = Or(x=w501, y=w502) -> (x .or. y?=w500:bool)
    n373 = feedback #18(-inf) -> (w521:dbl)
    n374 = Max & Min(x=w498, y=w521) -> (max(x,y)=w499:dbl)  [unwired: 1 out]
    n375 = feedback #19(-inf) -> (w515:dbl)
    n376 = Max & Min(x=w497, y=w515) -> (max(x,y)=w513:dbl)  [unwired: 1 out]
    n377 = Select(t=0.0, s=w504, f=w499) -> (s? t:f=w520:dbl)
    "Max Current (A)" <- w520
    n378 = feedback-in #18(w520) -> ()
    n379 = Select(t=0.0, s=w500, f=w513) -> (s? t:f=w514:dbl)
    "Max Total Current" <- w514
    n380 = feedback-in #19(w514) -> ()
    n381 = Greater?(x=w497, y="Current Tolerance") -> (0:w495:bool)
    n382 = shared-variable ".\\Voltage Reg.lvlib\\Above threshold voltage?"(w495) -> ()  [unwired: 1 in, 1 out]
  }
